vi "AO DM_WFS_master_v0.vi"() -> ()   [LabVIEW 2018]
uses:
  <userlib>/WaveKit.lib/Controls/Image information.ctl
  <userlib>/WaveKit.lib/Controls/Image general information.ctl
  <userlib>/WaveKit.lib/Controls/Image acquisition information.ctl
  <userlib>/WaveKit.lib/Controls/Point2D.ctl
  <userlib>/WaveKit.lib/Controls/Data alignment enum.ctl
  <userlib>/WaveKit.lib/Controls/StatisticsData.ctl
  <userlib>/WaveKit.lib/Controls/Wavefront Corrector states - ONE.ctl
  <userlib>/WaveKit.lib/Classes/Camera/Camera.lvclass
  <userlib>/WaveKit.lib/Classes/CameraSet/CameraSet.lvclass
  <userlib>/WaveKit.lib/Classes/Image/Image.lvclass
  <userlib>/WaveKit.lib/Classes/Phase/Phase.lvclass
  <userlib>/WaveKit.lib/Controls/HasoSlopes.lvclass
  <userlib>/WaveKit.lib/Controls/Pupil.lvclass
  <userlib>/WaveKit.lib/Classes/WavefrontCorrector/WavefrontCorrector.lvclass
  <userlib>/WaveKit.lib/Classes/WavefrontCorrectorSet/WavefrontCorrectorSet.lvclass
  <userlib>/WaveKit.lib/Classes/HasoEngine/HasoEngine.lvclass
  <userlib>/WaveKit.lib/Controls/SlopesEngineSetup.ctl
  <userlib>/WaveKit.lib/Controls/WavefrontReconstructionMode.ctl
  <vilib>/Utility/file.llb/Read From Spreadsheet File (DBL).vi
  <vilib>/Analysis/1siggen.llb/Ramp Pattern by Delta.vi
  <userlib>/WaveKit.lib/Classes/ModalCoef/ModalCoef.lvclass
  <vilib>/Analysis/NI_AALBase.lvlib
panel:
  in  "Device Status":enum32{"DM", "WFS", "Others"}(tab)
  out "DM Actuator Values":sgl[](graph)
  out "Initial State":T1[](array[typedef])
  out "ActuatorsNumber":i32
  out "Initial Positions":sgl[](array[numeric])
  out "Final Positions":sgl[](array[numeric])
  in  "Coef Min":dbl=-0.5 min=1.0
  in  "Coef Max":dbl=0.5 min=1.0
  out "Zernike Measured":dbl[](graph)
  out "Phase statistics":T2
  out "Phase values":sgl[][](graph)=[[nan, nan, nan, nan, nan, nan, nan, nan, nan, nan, nan, nan, nan, nan, nan, nan, nan, nan, nan, nan, nan, nan, nan, nan, nan, nan, nan, nan, nan, nan, nan, nan, nan, nan, nan, nan, nan, nan, nan, nan], [nan, nan, nan, nan, nan, nan, nan, nan, nan, nan, nan, nan, nan, nan, nan, nan, nan, nan, nan, nan, nan, nan, nan, nan, nan, nan, nan, nan, nan, nan, nan, nan, nan, nan, nan, nan, nan, nan, nan, nan], [nan, nan, nan, nan, nan, nan, nan, nan, nan, nan, nan, nan, nan, nan, nan, nan, nan, nan, nan, nan, nan, nan, nan, nan, nan, nan, nan, nan, nan, nan, nan, nan, nan, nan, nan, nan, nan, nan, nan, nan], [nan, nan, nan, nan, nan, nan, nan, nan, nan, nan, nan, nan, nan, nan, nan, nan, nan, nan, nan, nan, nan, nan, nan, nan, nan, nan, nan, nan, nan, nan, nan, nan, nan, nan, nan, nan, nan, nan, nan, nan], [nan, nan, nan, nan, nan, nan, nan, nan, nan, nan, nan, nan, nan, nan, -0.14441992, nan, 0.1501734, 0.22490476, 0.2674259, 0.28415325, 0.2792031, 0.2552752, 0.21375881, 0.15405469, nan, nan, nan, nan, nan, nan, nan, nan, nan, nan, nan, nan, nan, nan, nan, nan], [nan, nan, nan, nan, nan, nan, nan, nan, nan, nan, nan, nan, nan, nan, 0.19143742, 0.2795512, 0.33646506, 0.37099743, 0.3877919, 0.3894302, 0.37774685, 0.35447162, 0.3212538, 0.27904776, 0.22675864, 0.15897867, nan, nan, nan, nan, nan, nan, nan, nan, nan, nan, nan, nan, nan, nan], [nan, nan, nan, nan, nan, nan, nan, nan, nan, nan, nan, nan, nan, 0.22618562, 0.290776, 0.33285964, 0.36044422, 0.3767934, 0.38285175, 0.37884915, 0.3652757, 0.3433441, 0.3149789, 0.28229773, 0.2464756, 0.20580466, 0.15268901, 0.06923797, nan, nan, nan, nan, nan, nan, nan, nan, nan, nan, nan, nan], [nan, nan, nan, nan, nan, nan, nan, nan, nan, nan, nan, nan, 0.19992779, 0.24616541, 0.27565512, 0.29675642, 0.31222007, 0.32191983, 0.32467726, 0.31943765, 0.30597392, 0.2852214, 0.25927368, 0.2309889, 0.20308714, 0.17653626, 0.14795627, 0.10568966, 0.024115691, nan, nan, nan, nan, nan, nan, nan, nan, nan, nan, nan], [nan, nan, nan, nan, nan, nan, nan, nan, nan, nan, nan, 0.14862825, 0.18219855, 0.20114602, 0.21551609, 0.22862102, 0.24014233, 0.24817906, 0.2505626, 0.24567793, 0.23295718, 0.21313797, 0.18829979, 0.16161954, 0.1367108, 0.11633411, 0.10019377, 0.081457645, 0.04156301, -0.057204023, nan, nan, nan, nan, nan, nan, nan, nan, nan, nan], [nan, nan, nan, nan, nan, nan, nan, nan, nan, nan, 0.08899155, 0.117771566, 0.12948777, 0.13732892, 0.14631097, 0.15688494, 0.16728252, 0.17497937, 0.17758016, 0.17335457, 0.16157834, 0.14275661, 0.11873307, 0.09261118, 0.06834036, 0.04974218, 0.038678437, 0.031985473, 0.016725859, -0.03676957, nan, nan, nan, nan, nan, nan, nan, nan, nan, nan], [nan, nan, nan, nan, nan, nan, nan, nan, nan, nan, 0.058377307, 0.069048055, 0.0725615, 0.07683456, 0.0840318, 0.09335055, 0.10271386, 0.1097376, 0.11226265, 0.10867052, 0.09812171, 0.08078306, 0.058033932, 0.032565817, 0.008214329, -0.010712444, -0.020921554, -0.022825297, -0.02489755, -0.05023362, -0.14592764, nan, nan, nan, nan, nan, nan, nan, nan, nan], [nan, nan, nan, nan, nan, nan, nan, nan, nan, -0.0018393314, 0.018310271, 0.023098737, 0.024714457, 0.027986258, 0.033823933, 0.041292578, 0.048749834, 0.054400377, 0.056548227, 0.05374936, 0.04499338, 0.029967438, 0.009379062, -0.014759185, -0.03905803, -0.059140373, -0.070816256, -0.0724436, -0.06894927, -0.07806298, -0.1393881, nan, nan, nan, nan, nan, nan, nan, nan, nan], [nan, nan, nan, nan, nan, nan, nan, nan, nan, -0.03322208, -0.017045017, -0.0123043535, -0.010394985, -0.007970343, -0.0042642877, 0.0003761826, 0.005164365, 0.009095938, 0.010986101, 0.009512841, 0.0033822758, -0.008344227, -0.02579559, -0.047820807, -0.071688615, -0.09321856, -0.107681155, -0.11187886, -0.10789668, -0.10908524, -0.14891545, -0.29341945, nan, nan, nan, nan, nan, nan, nan, nan], [nan, nan, nan, nan, nan, nan, nan, nan, nan, nan, -0.043187555, -0.03622458, -0.033755217, -0.03278728, -0.03198469, -0.030707732, -0.028716512, -0.026208155, -0.023933899, -0.023217455, -0.025771504, -0.03328519, -0.04682974, -0.06620631, -0.08943447, -0.1126552, -0.13079928, -0.13944486, -0.13836564, -0.13734597, -0.16491348, -0.2807172, nan, nan, nan, nan, nan, nan, nan, nan], [nan, nan, nan, nan, nan, nan, nan, nan, -0.13038255, -0.08328184, -0.060542934, -0.050779276, -0.048053104, -0.048984695, -0.05126809, -0.053124577, -0.05330209, -0.051303368, -0.04760214, -0.04368073, -0.041799206, -0.04448101, -0.05377527, -0.07043236, -0.09320336, -0.118551016, -0.14113419, -0.15550357, -0.15952203, -0.16009864, -0.18189941, -0.27977645, nan, nan, nan, nan, nan, nan, nan, nan], [nan, nan, nan, nan, nan, nan, nan, nan, -0.15416794, -0.09987456, -0.07151361, -0.05893044, -0.056102008, -0.058817875, -0.063637674, -0.067669004, -0.06878706, -0.06599128, -0.059670344, -0.051622536, -0.044753395, -0.042448726, -0.04769562, -0.062100213, -0.08502676, -0.11315687, -0.14084403, -0.16171429, -0.1720384, -0.17647736, -0.19687745, -0.284868, -0.53908885, -1.12795, nan, nan, nan, nan, nan, nan], [nan, nan, nan, nan, nan, nan, nan, nan, -0.17633308, -0.1131372, -0.07876157, -0.06330658, -0.060116876, -0.063924976, -0.07015394, -0.07493687, -0.07548633, -0.07052183, -0.060539607, -0.047784284, -0.035856243, -0.028966732, -0.030924596, -0.044017438, -0.06802279, -0.099662215, -0.13288532, -0.16044727, -0.17731819, -0.18653797, -0.20820689, -0.29237592, -0.5366785, nan, nan, nan, nan, nan, nan, nan], [nan, nan, nan, nan, nan, nan, nan, nan, -0.19826387, -0.12505035, -0.08430402, -0.06564974, -0.061443567, -0.06527472, -0.07152294, -0.07554153, -0.07411167, -0.0658889, -0.05163869, -0.034133032, -0.017655006, -0.0071354215, -0.007018423, -0.020031396, -0.046107426, -0.08178567, -0.12048963, -0.15415914, -0.17678727, -0.19048853, -0.21480094, -0.2999987, -0.54526997, nan, nan, nan, nan, nan, nan, nan], [nan, nan, nan, nan, nan, nan, nan, nan, -0.2214154, -0.13693352, -0.08914254, -0.06661926, -0.06048554, -0.06317037, -0.0681367, -0.07015528, -0.065784656, -0.053790003, -0.035310905, -0.013662348, 0.0062713036, 0.01901285, 0.01972933, 0.005542416, -0.023349542, -0.06307545, -0.10643376, -0.14466219, -0.17119798, -0.18806857, -0.21562657, -0.30642, -0.5640642, nan, nan, nan, nan, nan, nan, nan], [nan, nan, nan, nan, nan, nan, nan, nan, -0.24718054, -0.14940841, -0.093277775, -0.0658183, -0.056708053, -0.05720259, -0.059951056, -0.05929426, -0.051715773, -0.036192447, -0.014265999, 0.010266874, 0.032073133, 0.04536258, 0.04520398, 0.028878966, -0.0030008797, -0.045963787, -0.092160165, -0.13235793, -0.16002774, -0.17817038, -0.20961209, -0.31157303, -0.5953845, nan, nan, nan, nan, nan, nan, nan], [nan, nan, nan, nan, nan, nan, nan, nan, -0.27748746, -0.16290864, -0.09610232, -0.062047683, -0.048735943, -0.04617936, -0.046241976, -0.042900223, -0.03261665, -0.014586102, 0.009311387, 0.03494107, 0.05674191, 0.068891875, 0.0666744, 0.04783368, 0.0136316735, -0.030755527, -0.0769404, -0.115639456, -0.14119013, -0.15893419, -0.19620675, -0.31774768, nan, nan, nan, nan, nan, nan, nan, nan], [nan, nan, nan, nan, nan, nan, nan, nan, -0.31623095, -0.17884897, -0.09729818, -0.0539262, -0.03469713, -0.028198741, -0.025418447, -0.019910373, -0.008048305, 0.010862423, 0.034768496, 0.05942371, 0.07931873, 0.0889112, 0.08400761, 0.06307276, 0.028166434, -0.014867521, -0.057410896, -0.09080534, -0.111413695, -0.12868427, -0.17697167, -0.3319423, nan, nan, nan, nan, nan, nan, nan, nan], [nan, nan, nan, nan, nan, nan, nan, nan, nan, -0.20170604, -0.09850275, -0.0411539, -0.0131010795, -0.0011654077, 0.0047943285, 0.01185911, 0.023955166, 0.041901454, 0.06374147, 0.08542206, 0.1018104, 0.10796184, 0.10047772, 0.0787158, 0.04554086, 0.007227666, -0.027947046, -0.052963093, -0.06777905, -0.08820889, -0.15871821, nan, nan, nan, nan, nan, nan, nan, nan, nan], [nan, nan, nan, nan, nan, nan, nan, nan, nan, -0.24239759, -0.10614249, -0.026831074, 0.015322472, 0.03581071, 0.046350636, 0.05505173, 0.06651187, 0.08204405, 0.10016226, 0.11737824, 0.12928592, 0.13183476, 0.12261822, 0.10192663, 0.073240966, 0.042765103, 0.017522467, 0.0014635092, -0.0110412, -0.045025453, -0.15884721, nan, nan, nan, nan, nan, nan, nan, nan, nan], [nan, nan, nan, nan, nan, nan, nan, nan, nan, nan, -0.13597216, -0.021381527, 0.04426403, 0.07956008, 0.09847209, 0.110732496, 0.122154154, 0.13505057, 0.14887714, 0.16113368, 0.16849175, 0.16803522, 0.1584293, 0.14075197, 0.118653886, 0.09743117, 0.0815231, 0.06987105, 0.048498146, -0.020404778, nan, nan, nan, nan, nan, nan, nan, nan, nan, nan], [nan, nan, nan, nan, nan, nan, nan, nan, nan, nan, nan, -0.04876471, 0.05625415, 0.117832564, 0.15310521, 0.17423762, 0.18897903, 0.20128381, 0.21210447, 0.22038196, 0.22418612, 0.221881, 0.21311647, 0.19937092, 0.1836943, 0.16922635, 0.15598845, 0.13537171, 0.081669986, nan, nan, nan, nan, nan, nan, nan, nan, nan, nan, nan], [nan, nan, nan, nan, nan, nan, nan, nan, nan, nan, nan, nan, 0.014031529, 0.121263236, 0.18738765, 0.22803904, 0.25380248, 0.2710389, 0.28282017, 0.2899857, 0.29225817, 0.2892868, 0.28139976, 0.26978248, 0.25571787, 0.23844866, 0.21115, 0.15442081, nan, nan, nan, nan, nan, nan, nan, nan, nan, nan, nan, nan], [nan, nan, nan, nan, nan, nan, nan, nan, nan, nan, nan, nan, nan, nan, 0.15212902, 0.2306162, 0.28129596, 0.31381333, 0.33402625, 0.3450995, 0.34855807, 0.34515002, 0.33529556, 0.31882071, 0.29360068, 0.25266168, nan, nan, nan, nan, nan, nan, nan, nan, nan, nan, nan, nan, nan, nan], [nan, nan, nan, nan, nan, nan, nan, nan, nan, nan, nan, nan, nan, nan, nan, nan, 0.1979487, 0.2623494, 0.30271748, 0.32490522, 0.33223343, 0.3261181, 0.30614072, 0.26925305, nan, nan, nan, nan, nan, nan, nan, nan, nan, nan, nan, nan, nan, nan, nan, nan], [nan, nan, nan, nan, nan, nan, nan, nan, nan, nan, nan, nan, nan, nan, nan, nan, nan, nan, nan, nan, nan, nan, nan, nan, nan, nan, nan, nan, nan, nan, nan, nan, nan, nan, nan, nan, nan, nan, nan, nan], [nan, nan, nan, nan, nan, nan, nan, nan, nan, nan, nan, nan, nan, nan, nan, nan, nan, nan, nan, nan, nan, nan, nan, nan, nan, nan, nan, nan, nan, nan, nan, nan, nan, nan, nan, nan, nan, nan, nan, nan], [nan, nan, nan, nan, nan, nan, nan, nan, nan, nan, nan, nan, nan, nan, nan, nan, nan, nan, nan, nan, nan, nan, nan, nan, nan, nan, nan, nan, nan, nan, nan, nan, nan, nan, nan, nan, nan, nan, nan, nan]] caption="Wavefront"
  out "HASO intensity":u32[][](graph)
  out "Current error":errorcluster
  out "Output path":path=path "D:/Data"
  in  "Current status":string="Test1"
  out "HASO ready":bool
  in  "Live Wavefront":bool
  in  "Update DM":bool
  in  "Tab Control":T3(tab)
  in  "Initial haso file":path=path "D:/SystemAlignment/system_aberration_residual_20200816.has"
  in  "interaction matrix file":path=path "D:/SystemAlignment/IM_20200807_1p5s.aomi"
  in  "DM configuration file":path=path "C:/Program Files (x86)/Imagine Optic/Configuration Files/WaveFrontCorrector_mirao52-e_0326.dat"
  in  "Haso configuration file":path=path "C:/Program Files (x86)/Imagine Optic/Configuration Files/HASO3_first_7364.dat"
  in  "Coef value":dbl=0.5 min=1.0
  in  "Idx end":u32=20 min=1
  in  "Idx start":u32=1 min=1
  in  "Subfolder":string="Test1"
  in  "Folder Name":string="Test"
  in  "Record Response":bool
  in  "Net Rp":bool
  in  "Input type":T4(ring)=enum."Zernike Coef"
  in  "Additional Command":bool=TRUE
  in  "Offset command file":path=path "D:/SystemAlignment/system_aberration_20200627.dat"
  in  "Initial offset":bool=TRUE
  in  "Additional file":path=path "D:/SystemAlignment/system_aberration_20191029.dat"
  out "Zern coef out":sgl[](array[numeric])
  out "Zern index out":i32[](array[numeric])
  in  "Zern index in":i32[](array[numeric])
  in  "Zern coef in":sgl[](array[numeric])
  in  "idxType":enum16{"Wyant", "ANSI"}(ring)
  in  "Filter":u8[](array[numeric])
  out "exposure_duration_us (get)":u32
  in  "exposure_duration_s (set)":dbl=0.5 min=1.0
  out "nb_images (get)":u32=10
  in  "nb_images (set)":u32=1 min=1
  in  "Save File":bool
  in  "File Base Name":string="Test"
  in  "Main Path":path=path "D:/Data"
  in  "Record Batch":bool
  out "Acquisition information":T5={"Image general information"={"Camera serial number"="", "Smearing removed"=FALSE, "Background image removed"=FALSE, "Time Stamp"=timestamp(0 s since 1904-01-01), "Comment"="", "Camera_MAX_Level"=0}, "Acquisition information"={"Exposure duration (us)"=0, "Exposure duration specified (us)"=0, "Gain"=0.0, "Number of summed images"=0, "Trigger type"=""}, "Number of pixels"={"X"=0, "Y"=0}, "Number of bits"=enum."16"}
  in  "Init":bool
  in  "Reset error":bool
  in  "Exit":bool
  in  "Stop HASO":bool
  in  "Start HASO":bool
  # "AO DM_WFS_master_v0.vi: (last update: 20200817)\nControl deformable mirror and wavefront sensor, check DM response be WFS \n1, Record DM response;\n2, Test DM response to single Zernike component in batch"
  # "um"
  # "HASO Parameters"
  # "Check DM Response"
  # "Need to turn OFF live wavefront"
  # "Batch range"
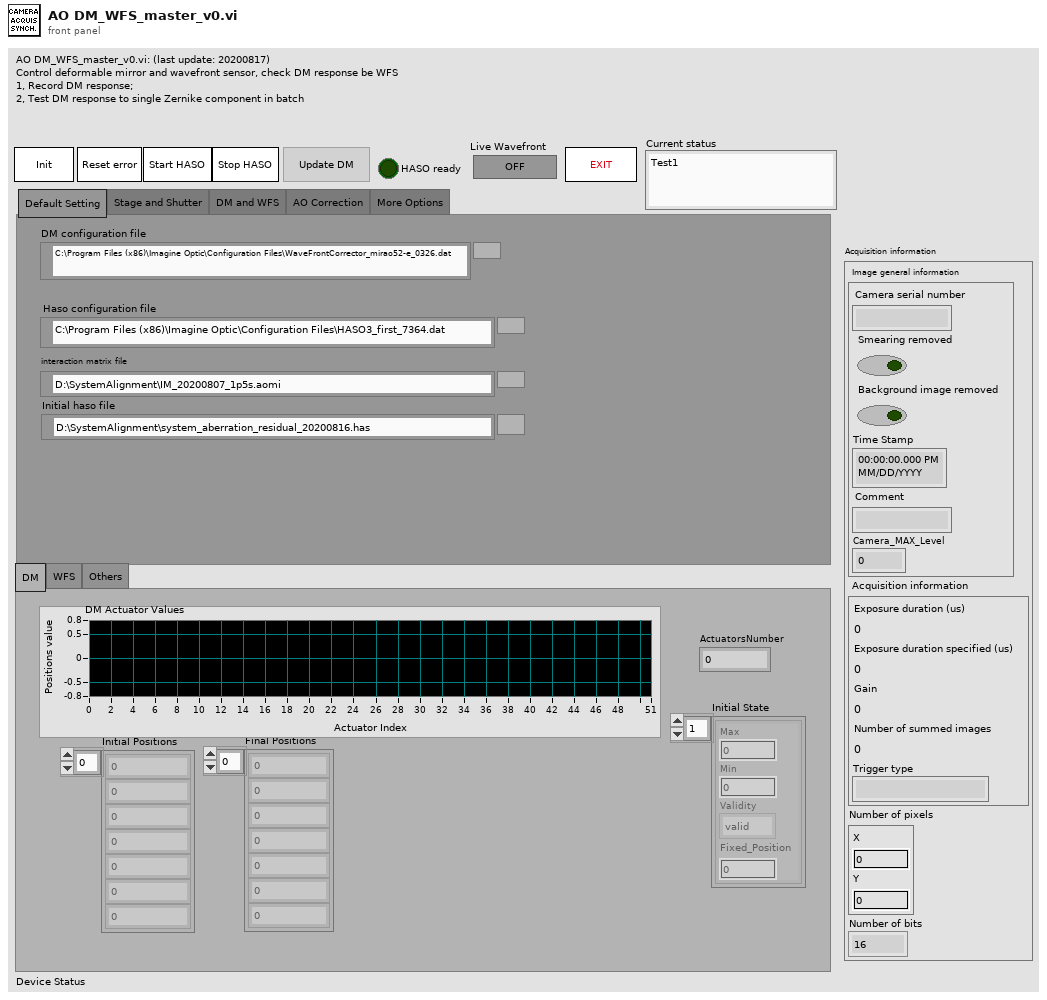
[diagram p1: front panel]
types:
  T1 = typedef "Wavefront Corrector states - ONE.ctl" = cluster{"Max":sgl, "Min":sgl, "Validity":enum16{"valid", "fixed", "invalid"}, "Fixed_Position":sgl}
  T2 = typedef "StatisticsData.ctl" = cluster{"PV":sgl, "RMS":dbl, "Max":sgl, "Min":sgl}
  T3 = enum32{"Default Setting", "Stage and Shutter", "DM and WFS", "AO Correction", "More Options"}
  T4 = enum16{"Zero Input", "Command File", "Zernike Coef", "Zernike File"}
  T5 = typedef "Image information.ctl" = cluster{"Image general information":T6, "Acquisition information":T7, "Number of pixels":T8, "Number of bits":T9}
  T6 = typedef "Image general information.ctl" = cluster{"Camera serial number":string, "Smearing removed":bool, "Background image removed":bool, "Time Stamp":timestamp, "Comment":string, "Camera_MAX_Level":i32}
  T7 = typedef "Image acquisition information.ctl" = cluster{"Exposure duration (us)":i32, "Exposure duration specified (us)":i32, "Gain":sgl, "Number of summed images":i32, "Trigger type":string}
  T8 = typedef "Point2D.ctl" = cluster{"X":u32, "Y":u32}
  T9 = typedef "Data alignment enum.ctl" = enum16{"8", "16", "32"}
  T10 = typedef "SlopesEngineSetup.ctl" = cluster{"Start sub-aperture":T8, "Pupil average":dbl}
  T11 = typedef "CameraSpecifications.ctl" = cluster{"Grabber name":string, "Camera name":string, "Camera sn":string, "Pixels_um":T12, "Maximum level":u32, "Data alignment":T9, "Is signed":bool, "Acquisition start":T8, "Acquisition length":T8, "MaxFrameRate_Hz":sgl, "Chip type":enum16{"Progressive scan", "Frame transfert"}}
  T12 = typedef "General dimensions definition.ctl" = cluster{"Size":T8, "Step":T13}
  T13 = typedef "Point2Df.ctl" = cluster{"X":sgl, "Y":sgl}
  T14 = typedef "Wavefront Corrector Position.ctl" = sgl[]
  T15 = typedef "WavefrontReconstructionMode.ctl" = enum16{"None", "Modal_Legendre", "Modal_Zernike", "Zonal", "Modal_Zonal_Zernike", "Modal_Zonal_Legendre"}
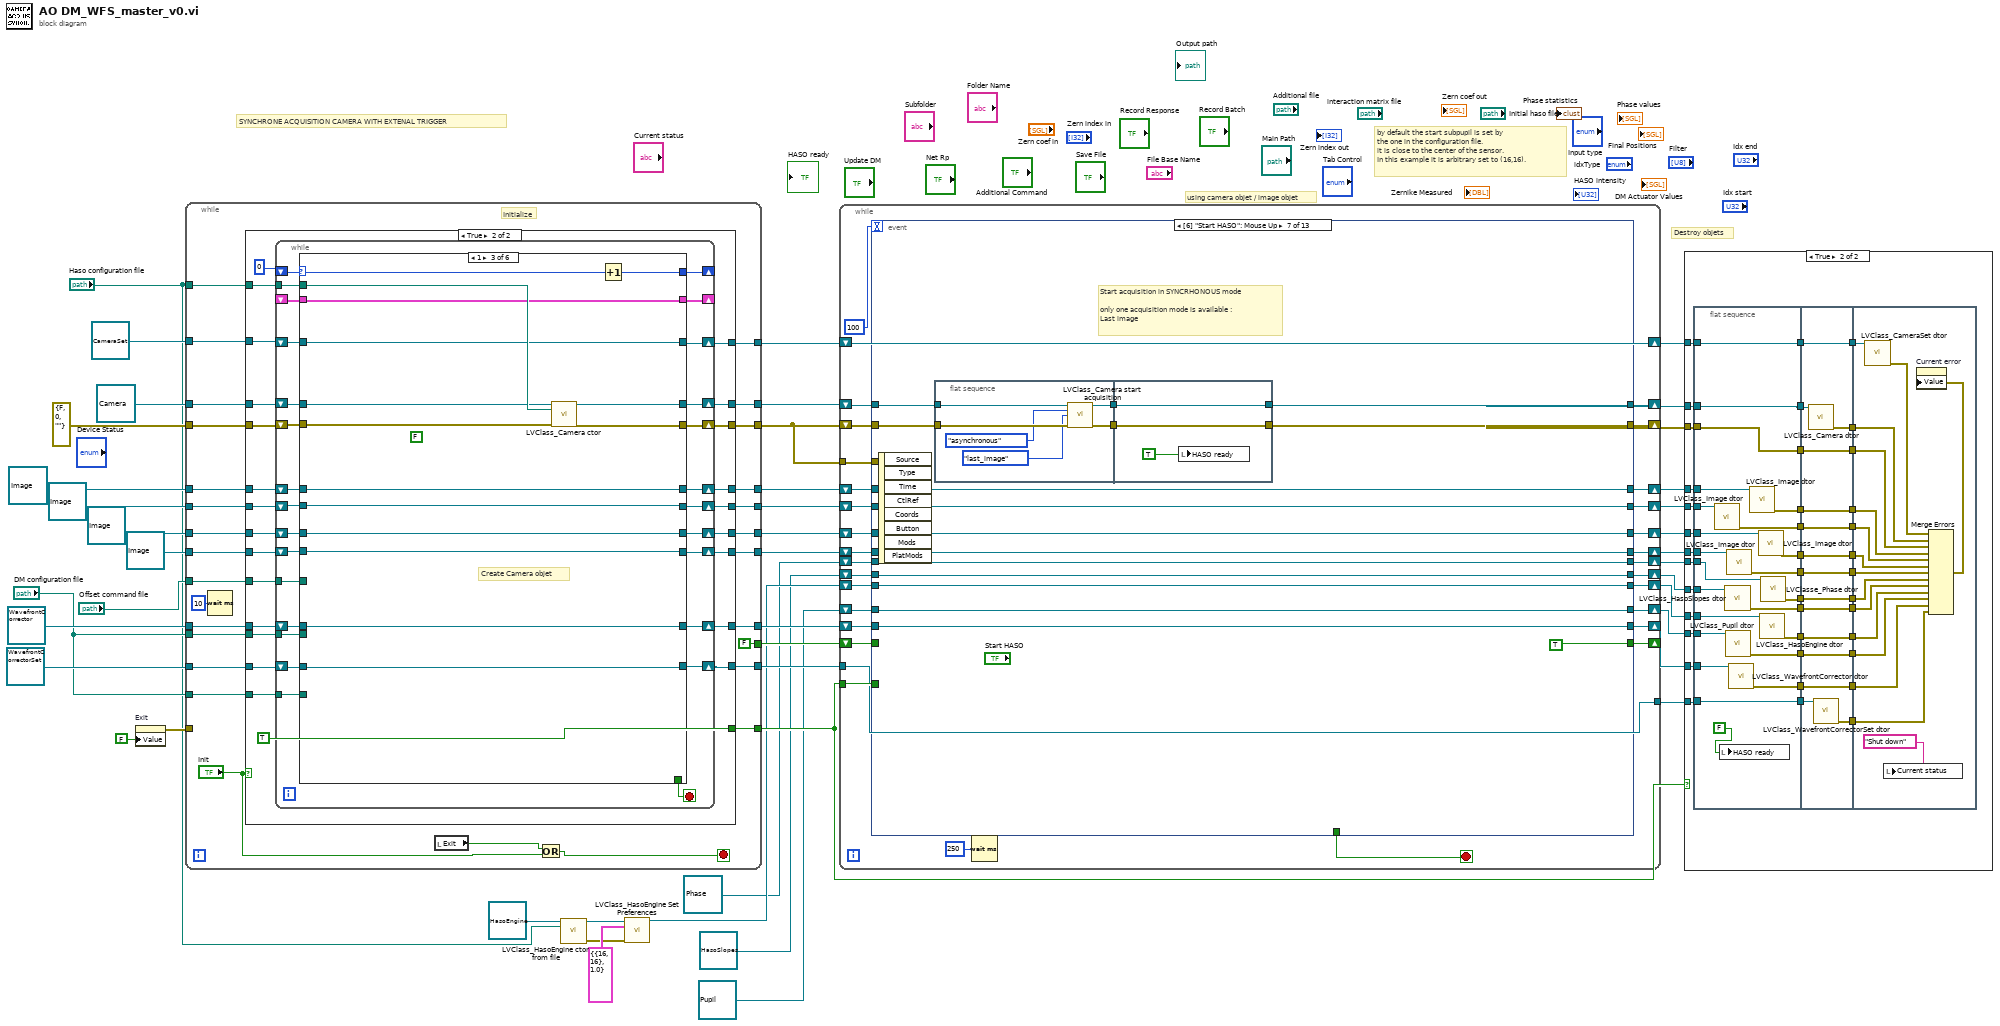
[diagram p0: block diagram]
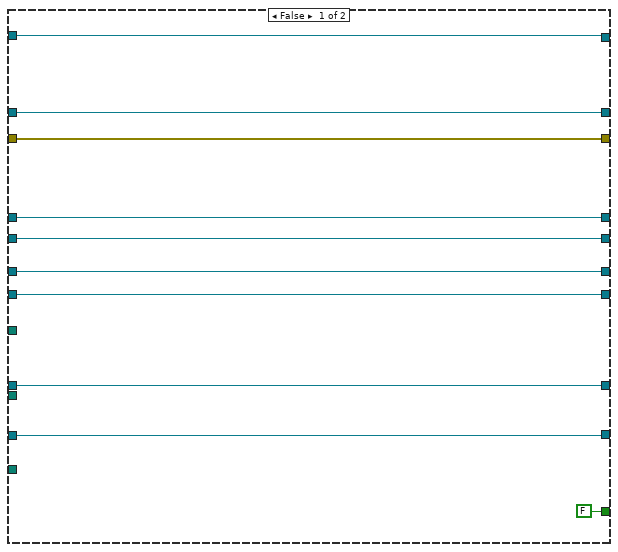
[diagram p3: hidden frame]
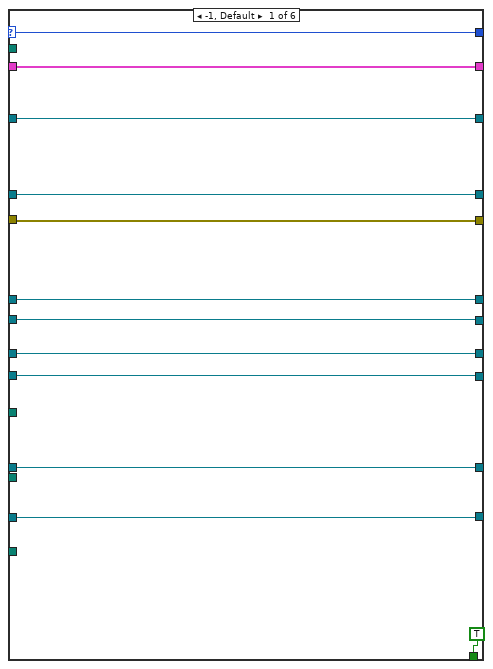
[diagram p4: hidden frame]
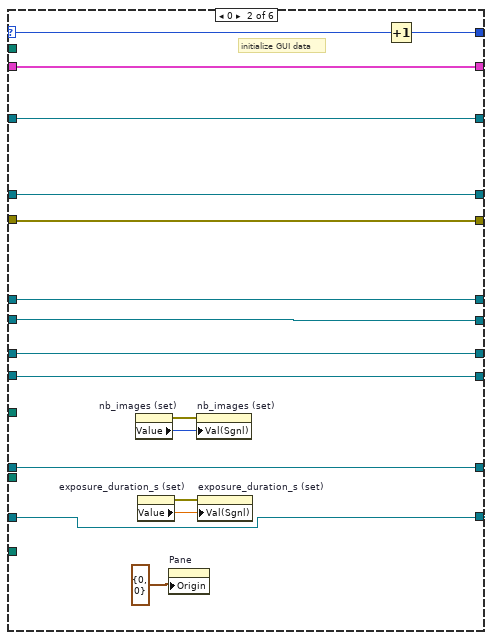
[diagram p5: hidden frame]
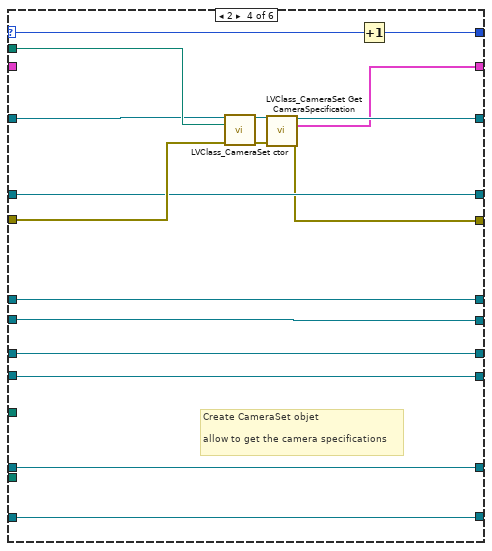
[diagram p6: hidden frame]
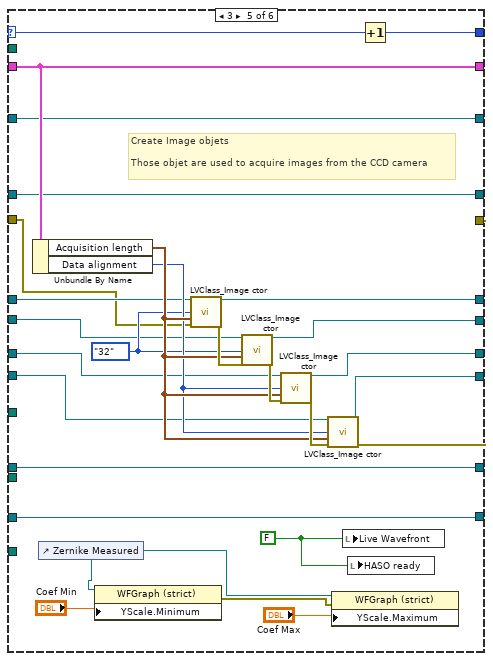
[diagram p7: hidden frame]
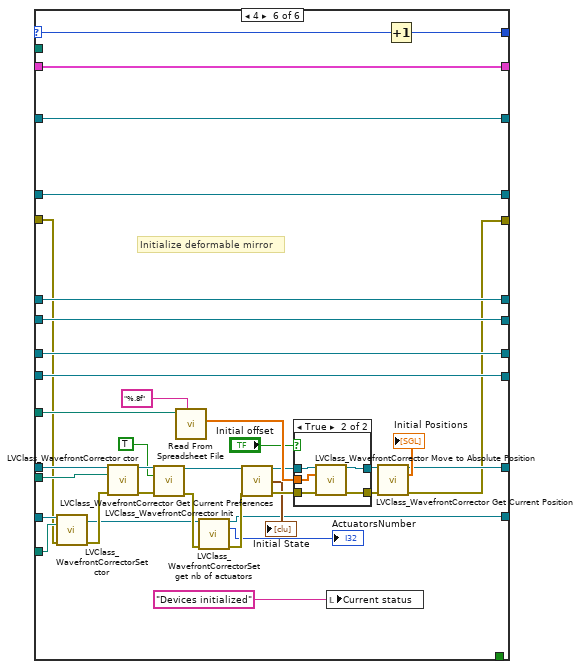
[diagram p8: hidden frame]
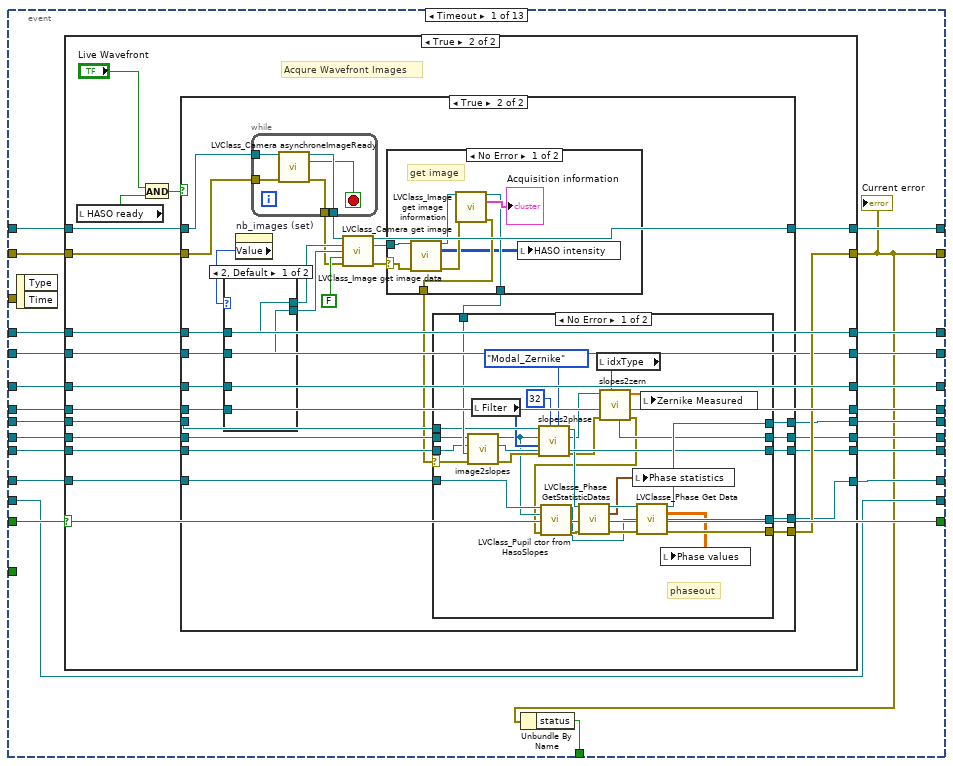
[diagram p10: hidden frame]
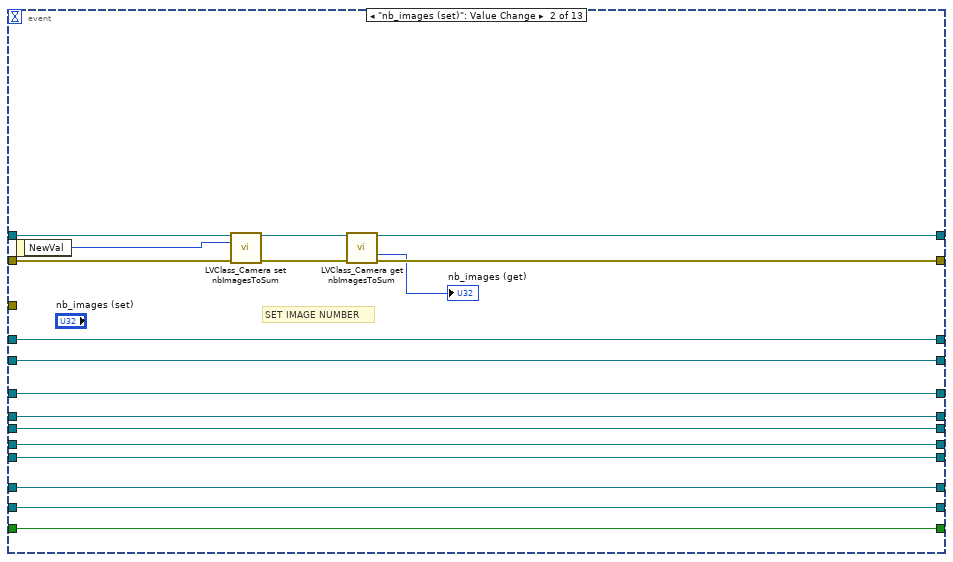
[diagram p16: hidden frame]
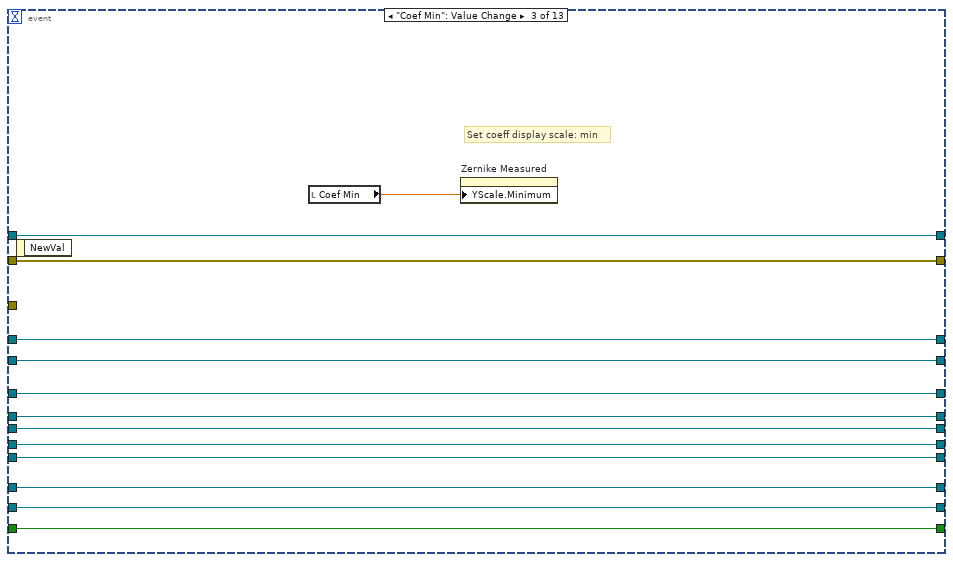
[diagram p17: hidden frame]
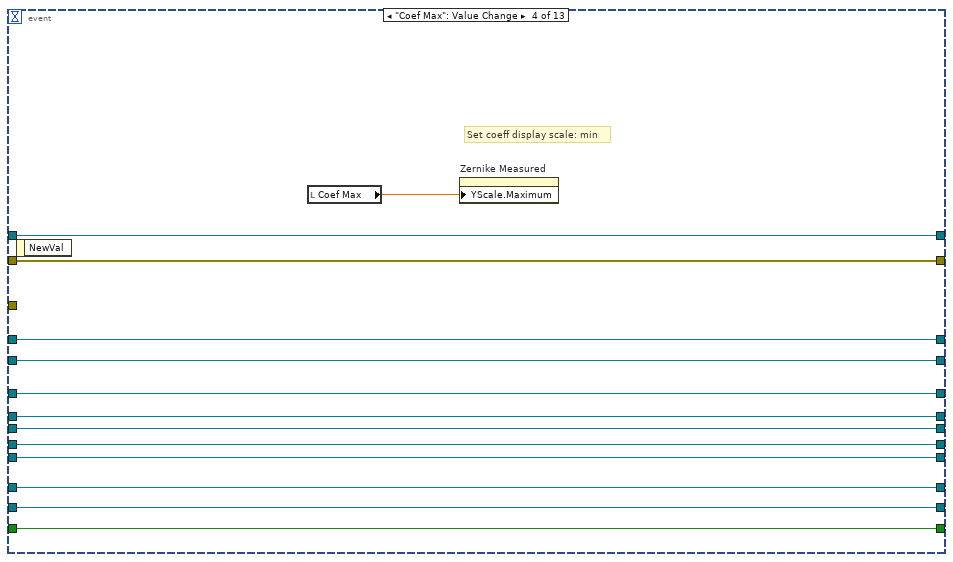
[diagram p18: hidden frame]
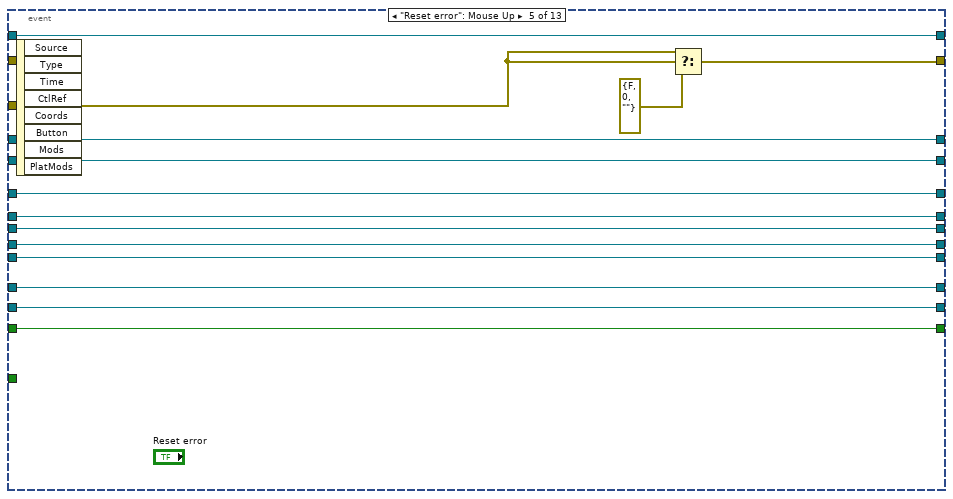
[diagram p19: hidden frame]
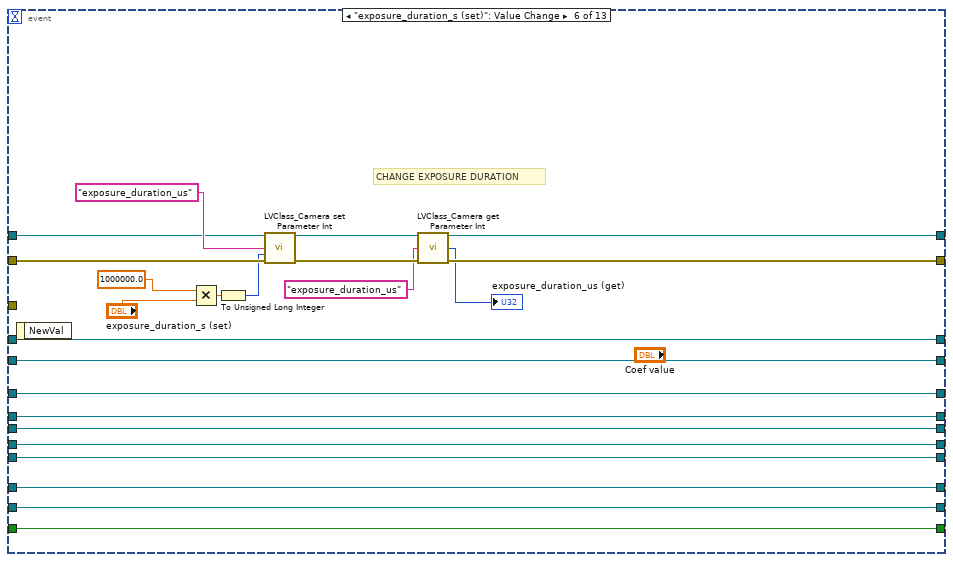
[diagram p20: hidden frame]
diagram:
  # "by default the start subpupil is set by \nthe one in the configuration file. \nit is close to the center of the sensor.\nIn this example it is arbitrary set to (16,16)."
  # "Destroy objets"
  # "using camera objet / image objet"
  # "SYNCHRONE ACQUISITION CAMERA WITH EXTENAL TRIGGER"
  n1 = property on="Exit" class="Bool (strict)"("Value"=FALSE ("Exit")) -> (error out=w22:errorcluster)  [unwired: 2 in, 1 out]
  n2 = while {
    tunnel: [FALSE] -> w39
    tunnel: [w73] -> w38
    tunnel: [w72] -> w37
    tunnel: [w71] -> w36
    tunnel: [w70] -> w35
    tunnel: [w69] -> w34
    tunnel: [w68] -> w33
    tunnel: refnum<class "Camera.lvclass"> refnum ("Camera.lvclass") -> [w67]
    tunnel: refnum<class "CameraSet.lvclass"> refnum ("CameraSet.lvclass") -> [w66]
    tunnel: refnum<class "Image.lvclass"> refnum ("Image in") -> [w65]
    tunnel: refnum<class "Image.lvclass"> refnum ("Image in") -> [w64]
    tunnel: refnum<class "Image.lvclass"> refnum ("Image in") -> [w63]
    tunnel: refnum<class "Image.lvclass"> refnum ("Image in") -> [w62]
    tunnel: errorcluster {"status"=FALSE, "code"=0, "source"=""} ("error out") -> [w61]
    tunnel: [w60] -> w25
    tunnel: [w58] -> w24
    tunnel: w22 -> [_]
    tunnel: "Haso configuration file" -> [w54]
    tunnel: "Offset command file" -> [w53]
    tunnel: refnum<class "WavefrontCorrectorSet.lvclass"> refnum ("WavefrontCorrectorSet in") -> [w52]
    tunnel: "DM configuration file" -> [w51]
    tunnel: refnum<class "WavefrontCorrector.lvclass"> refnum ("WavefrontCorrector in") -> [w50]
    tunnel: "DM configuration file" -> [w49]
    tunnel: [w48] -> w17
    tunnel: [w47] -> w16
    stop <- w55 stop-if-true
    # "Initialize"
    n3 = Wait (ms)(milliseconds to wait=u32 10) -> ()  [unwired: 1 out]
    n4 = case shown="True" "Init" {
      tunnel: [w84 w108] -> w73
      tunnel: [w83 w107] -> w72
      tunnel: [w81 w106] -> w71
      tunnel: [w80 w105] -> w70
      tunnel: [w79 w104] -> w69
      tunnel: [w78 w103] -> w68
      tunnel: w67 -> [w84 w102]
      tunnel: w66 -> [w83 w100]
      tunnel: w65 -> [w81 w99]
      tunnel: w64 -> [w80 w98]
      tunnel: w63 -> [w79 w97]
      tunnel: w62 -> [w78 w96]
      tunnel: w61 -> [w82 w95]
      tunnel: [w82 w94] -> w60
      tunnel: [FALSE TRUE] -> w58
      tunnel: w54 -> [_ w92]
      tunnel: w53 -> [_ w91]
      tunnel: w52 -> [w75 w85]
      tunnel: w51 -> [_ w90]
      tunnel: w50 -> [w76 w86]
      tunnel: w49 -> [_ w89]
      tunnel: [w76 w88] -> w48
      tunnel: [w75 w87] -> w47
      frame False {
      }
      frame True {
        n5 = while {
          tunnel: w92 -> [w133]
          shift-right: [w135] -> w108
          shift-left: w102 -> [w127]
          shift-right: [w117] -> _
          shift-left: 0 -> [w116]
          shift-right: [w134] -> w107
          shift-left: w100 -> [w126]
          shift-right: [w125] -> _
          shift-left: _ -> [w123]
          shift-right: [w132] -> w106
          shift-left: w99 -> [w124]
          shift-right: [w131] -> w105
          shift-left: w98 -> [w122]
          shift-right: [w130] -> w104
          shift-left: w97 -> [w120]
          shift-right: [w129] -> w103
          shift-left: w96 -> [w121]
          shift-right: [w128] -> w94
          shift-left: w95 -> [w118]
          tunnel: w91 -> [w115]
          tunnel: w90 -> [w114]
          tunnel: w89 -> [w113]
          shift-right: [w112] -> w88
          shift-left: w86 -> [w110]
          shift-right: [w111] -> w87
          shift-left: w85 -> [w109]
          stop <- w119 stop-if-true
          n6 = case shown="1" w116 {
            tunnel: [w147 w151 w179 w189 w211 w261] -> w135
            tunnel: w133 -> [_ _ w178 w193 _ _]
            tunnel: [w146 w155 w176 w194 w212 w260] -> w134
            tunnel: [w139 w156 w170 w184 w218 w255] -> w132
            tunnel: [w140 w157 w171 w185 w217 w256] -> w131
            tunnel: [w141 w158 w172 w186 w216 w257] -> w130
            tunnel: [w142 w159 w173 w187 w215 w258] -> w129
            tunnel: [w143 w150 w175 w188 w214 w229] -> w128
            selector: w116 -> [w138 w153 w168 w183 w206 w227]
            tunnel: w127 -> [w147 w151 w177 w189 w211 w261]
            tunnel: w126 -> [w146 w155 w176 w192 w212 w260]
            tunnel: [w144 w152 w174 w191 w213 w259] -> w125
            tunnel: w124 -> [w139 w156 w170 w184 w210 w255]
            tunnel: w123 -> [w144 w152 w174 _ w213 w259]
            tunnel: w122 -> [w140 w157 w171 w185 w209 w256]
            tunnel: w121 -> [w142 w159 w173 w187 w208 w258]
            tunnel: w120 -> [w141 w158 w172 w186 w207 w257]
            tunnel: [TRUE _ _ _ _ _] -> w119
            tunnel: w118 -> [w143 w150 w167 w190 w204 w230]
            tunnel: [w138 w154 w169 w182 w205 w226] -> w117
            tunnel: w115 -> [_ _ _ _ _ w237]
            tunnel: w109 -> [w136 w148 w165 w180 w202 w235]
            tunnel: w114 -> [_ _ _ _ _ w234]
            tunnel: w110 -> [w137 w149 w166 w181 w203 w233]
            tunnel: w113 -> [_ _ _ _ _ w232]
            tunnel: [w137 w149 w166 w181 w203 w231] -> w112
            tunnel: [w136 w148 w165 w180 w202 w228] -> w111
            frame -1, Default {
            }
            frame 0 {
              # "initialize GUI data"
              n7 = property on="nb_images (set)" class="DigNum (strict)"() -> (error out=w164:errorcluster, "Value"=w163:u32)  [unwired: 2 in, 1 out]
              n8 = property on="exposure_duration_s (set)" class="DigNum (strict)"() -> (error out=w160:errorcluster, "Value"=w162:dbl)  [unwired: 2 in, 1 out]
              n9 = property on="Pane" class="Pane"("Origin"=cluster{"Horizontal":i16, "Vertical":i16} {"Horizontal"=0, "Vertical"=0} ("Front Panel Window:Origin")) -> ()  [unwired: 2 in, 2 out]
              n10 = property on="nb_images (set)" class="DigNum (strict)"(error in=w164, "Val(Sgnl)"=w163) -> ()  [unwired: 1 in, 2 out]
              n11 = property on="exposure_duration_s (set)" class="DigNum (strict)"(error in=w160, "Val(Sgnl)"=w162) -> ()  [unwired: 1 in, 2 out]
              n12 = Increment(x=w153) -> (x+1=w154:i32)
            }
            frame 1 {
              (unwired) FALSE ("Acq required")
              # "Create Camera objet"
              n13 = call <userlib>:"LVClass_Camera ctor.vi"("Camera"=w177, "Configuration file path"=w178, "error in (no error)"=w167) -> ("Camera (new)"=w179:refnum<class "Camera.lvclass">, "error out"=w175:errorcluster)  [unwired: 11 in]
              n14 = Increment(x=w168) -> (x+1=w169:i32)
            }
            frame 2 {
              # "Create CameraSet objet\n\nallow to get the camera specifications"
              n15 = call <userlib>:"LVClass_CameraSet ctor.vi"("CameraSet.lvclass"=w192, "Configuration file path"=w193, "error in (no error)"=w190) -> ("CameraSet.lvclass"=w196:refnum<class "CameraSet.lvclass">, "error out"=w195:errorcluster)  [unwired: 11 in]
              n16 = call <userlib>:"LVClass_CameraSet Get CameraSpecification.vi"("CameraSet.lvclass"=w196, "error in (no error)"=w195) -> ("CameraSet.lvclass"=w194:refnum<class "CameraSet.lvclass">, "Camera Config"=w191:T11, "error out"=w188:errorcluster)  [unwired: 11 in]
              n17 = Increment(x=w183) -> (x+1=w182:i32)
            }
            frame 3 {
              w201 = FALSE
              w219 = Data_alignment_enum."32" ("Data alignment")
              # "Create Image objets\n\nThose objet are used to acquire images from the CCD camera"
              n18 = Unbundle By Name(w213) -> ("Acquisition length"=w221:T8, "Data alignment"=w220:T9)
              n19 = control-ref of="Zernike Measured"() -> (w198:refnum<vi>)
              n20 = property on="Property Node" class="WFGraph (strict)"(reference=w198, "YScale.Minimum"="Coef Min") -> (error out=w197:errorcluster)  [unwired: 1 in, 1 out]
              n21 = call <userlib>:"LVClass_Image ctor.vi"("Image in"=w210, "Data alignment"=w219, "Size"=w221, "error in (no error)"=w204) -> ("Image out"=w218:refnum<class "Image.lvclass">, "error out"=w222:errorcluster)  [unwired: 10 in]
              n22 = call <userlib>:"LVClass_Image ctor.vi"("Image in"=w209, "Data alignment"=w219, "Size"=w221, "error in (no error)"=w222) -> ("Image out"=w217:refnum<class "Image.lvclass">, "error out"=w223:errorcluster)  [unwired: 10 in]
              n23 = call <userlib>:"LVClass_Image ctor.vi"("Image in"=w207, "Data alignment"=w220, "Size"=w221, "error in (no error)"=w223) -> ("Image out"=w216:refnum<class "Image.lvclass">, "error out"=w224:errorcluster)  [unwired: 10 in]
              n24 = call <userlib>:"LVClass_Image ctor.vi"("Image in"=w208, "Data alignment"=w220, "Size"=w221, "error in (no error)"=w224) -> ("Image out"=w215:refnum<class "Image.lvclass">, "error out"=w214:errorcluster)  [unwired: 10 in]
              n25 = property on="Property Node" class="WFGraph (strict)"(reference=w198, error in=w197, "YScale.Maximum"="Coef Max") -> ()  [unwired: 2 out]
              n26 = local write "Live Wavefront"(w201) -> ()
              n27 = local write "HASO ready"(w201) -> ()
              n28 = Increment(x=w206) -> (x+1=w205:i32)
            }
            frame 4 {
              (unwired) "DM "
              (unwired) "DM "
              # "Initialize deformable mirror"
              n29 = call <userlib>:"LVClass_WavefrontCorrectorSet ctor.vi"("WavefrontCorrectorSet in"=w235, "PathToWavefrontCorrectorSetupFile"=w234, "error in (no error)"=w230) -> ("WavefrontCorrectorSet out"=w242:refnum<class "WavefrontCorrectorSet.lvclass">, "error out"=w251:errorcluster)  [unwired: 11 in]
              n30 = call <userlib>:"LVClass_WavefrontCorrector ctor.vi"("WavefrontCorrector in"=w233, "PathToWavefrontCorrectorSetupFile"=w232, "error in (no error)"=w251) -> ("WavefrontCorrector out"=w239:refnum<class "WavefrontCorrector.lvclass">, "error out"=w240:errorcluster)  [unwired: 11 in]
              n31 = call <userlib>:"LVClass_WavefrontCorrector Init.vi"("WavefrontCorrector in"=w239, "set_init_state_from_config_file"=TRUE, "error in (no error)"=w240) -> ("WavefrontCorrector out"=w243:refnum<class "WavefrontCorrector.lvclass">, "error out"=w252:errorcluster)  [unwired: 11 in]
              n32 = call-poly <vilib>:"Read From Spreadsheet File.vi"("format (%.3f)"="%.8f", "file path (dialog if empty)"=w237) -> ("first row"=w254:dbl[])  [unwired: 5 in, 4 out]
              n33 = call <userlib>:"LVClass_WavefrontCorrectorSet get nb of actuators.vi"("WavefrontCorrectorSet in"=w242, "error in (no error)"=w252) -> ("WavefrontCorrectorSet out"=w228:refnum<class "WavefrontCorrectorSet.lvclass">, "ActuatorsNumber"=→"ActuatorsNumber":i32, "error out"=w253:errorcluster)  [unwired: 11 in]
              n34 = call <userlib>:"LVClass_WavefrontCorrector Get Current Preferences.vi"("WavefrontCorrector in"=w243, "error in (no error)"=w253) -> ("WavefrontCorrector out"=w248:refnum<class "WavefrontCorrector.lvclass">, "Mirror preferences.Wavefront Corrector State"=→"Initial State":T1[], "error out"=w249:errorcluster)  [unwired: 10 in, 1 out]
              n35 = case shown="True" "Initial offset" {
                tunnel: w254 -> [_ w268]
                tunnel: [w263 w267] -> w246
                tunnel: [w262 w266] -> w247
                tunnel: w248 -> [w263 w265]
                tunnel: w249 -> [w262 w264]
                frame False {
                }
                frame True {
                  n36 = call <userlib>:"LVClass_WavefrontCorrector Move to Absolute Position.vi"("WavefrontCorrector in"=w265, "Absolute Positions"=w268, "error in (no error)"=w264) -> ("WavefrontCorrector out"=w267:refnum<class "WavefrontCorrector.lvclass">, "error out"=w266:errorcluster)  [unwired: 11 in]
                }
              }
              n37 = local write "Current status"("Devices initialized") -> ()
              n38 = call <userlib>:"LVClass_WavefrontCorrector Get Current Position.vi"("WavefrontCorrector in"=w246, "error in (no error)"=w247) -> ("WavefrontCorrector out"=w231:refnum<class "WavefrontCorrector.lvclass">, "Wavefront Corrector Position"=→"Initial Positions":T14, "error out"=w229:errorcluster)  [unwired: 11 in]
              n39 = Increment(x=w227) -> (x+1=w226:i32)
            }
          }
        }
      }
    }
    n40 = local read "Exit"() -> (w57:bool)
    n41 = Or(x=w57, y="Init") -> (x .or. y?=w55:bool)
  }
  n42 = call <userlib>:"LVClass_HasoEngine ctor from file.vi"("HasoEngine in"=refnum<class "HasoEngine.lvclass"> refnum, "Configuration file path"="Haso configuration file") -> ("HasoEngine out"=w13:refnum<class "HasoEngine.lvclass">, "error out"=w14:errorcluster)  [unwired: 12 in]
  n43 = call <userlib>:"LVClass_HasoEngine Set Preferences.vi"("HasoEngine in"=w13, "Slopes_HasoEngine_Setup"=T10 {"Start sub-aperture"={"X"=16, "Y"=16}, "Pupil average"=1.0}, "error in (no error)"=w14) -> ("HasoEngine out"=w10:refnum<class "HasoEngine.lvclass">)  [unwired: 11 in, 1 out]
  n44 = while {
    shift-right: [w296] -> w46
    shift-left: w25 -> [w298]
    shift-right: [w294] -> w45
    shift-left: w38 -> [w295]
    shift-right: [w288] -> w44
    shift-left: w36 -> [w293]
    shift-right: [w287] -> w43
    shift-left: w35 -> [w292]
    shift-right: [w286] -> w42
    shift-left: w34 -> [w291]
    shift-right: [w285] -> w41
    shift-left: w33 -> [w290]
    shift-right: [w284] -> _
    shift-left: w39 -> [w289]
    shift-right: [w283] -> w40
    shift-left: w37 -> [w283]
    tunnel: w25 -> [w282]
    tunnel: w24 -> [w281]
    tunnel: w16 -> [w270]
    shift-right: [w278] -> w9
    shift-left: refnum<class "HasoSlopes.lvclass"> refnum ("HasoSlopes in") -> [w277]
    shift-right: [w276] -> w4
    shift-left: w10 -> [w279]
    shift-right: [w273] -> w5
    shift-left: refnum<class "Phase.lvclass"> refnum ("Phase in") -> [w275]
    shift-right: [w272] -> w3
    shift-left: refnum<class "Pupil.lvclass"> refnum ("Pupil in") -> [w274]
    tunnel: [w270] -> w2
    shift-right: [w269] -> w1
    shift-left: w17 -> [w271]
    stop <- w297 stop-if-true
    n45 = event shown="[6] \"Start HASO\": Mouse Up" {
      selector: _ -> [_ _ _ _ _ _ _ _ _ _ _ _ _]
      dyn-events: _ -> [_ _ _ _ _ _ _ _ _ _ _ _ _]
      timeout: 100 -> [_ _ _ _ _ _ _ _ _ _ _ _ _]
      tunnel: w298 -> [w314 w452 w455 w468 _ w515 w531 w549 w577 w668 w1191 _ w1731]
      tunnel: [w300 _ _ _ _ _ _ _ w578 w669 w1192 "Exit" TRUE ("Exit")] -> w297
      tunnel: [w301 w450 w455 w468 w486 w510 w529 w555 w576 w667 w1190 w1715 w1736] -> w296
      tunnel: w295 -> [w319 w451 w456 w469 w488 w514 w532 w556 w572 w656 w1179 w1716 w1738]
      tunnel: [w318 w449 w456 w469 w488 w511 w530 w557 w572 w656 w1179 w1714 w1737] -> w294
      tunnel: w293 -> [w322 w442 w463 w476 w490 w504 w527 w551 w588 w663 w1186 w1710 w1732]
      tunnel: w292 -> [w321 w443 w464 w477 w491 w505 w526 w552 w587 w662 w1185 w1711 w1733]
      tunnel: w291 -> [w320 w444 w465 w478 w492 w506 w525 w553 w586 w661 w1184 w1712 w1734]
      tunnel: w290 -> [w315 w445 w466 w479 w493 w507 w524 w554 w585 w660 w1183 w1713 w1735]
      tunnel: w289 -> [w311 w441 w462 w475 w489 w503 _ _ w573 w665 w1188 _ _]
      tunnel: [w317 w442 w463 w476 w490 w504 w527 w551 w588 w663 w1186 w1710 w1732] -> w288
      tunnel: [w316 w443 w464 w477 w491 w505 w526 w552 w587 w662 w1185 w1711 w1733] -> w287
      tunnel: [w313 w444 w465 w478 w492 w506 w525 w553 w586 w661 w1184 w1712 w1734] -> w286
      tunnel: [w312 w445 w466 w479 w493 w507 w524 w554 w585 w660 w1183 w1713 w1735] -> w285
      tunnel: [w311 w441 w462 w475 w489 w503 TRUE FALSE w573 w665 w1188 FALSE FALSE] -> w284
      tunnel: w282 -> [_ _ _ _ w485 _ _ _ _ _ _ _ _]
      tunnel: w281 -> [_ _ _ _ _ _ _ _ _ _ _ w1708 _]
      tunnel: w277 -> [w310 w439 w460 w473 w483 w497 w522 w547 w569 w658 w1181 w1706 w1728]
      tunnel: w279 -> [w309 w438 w459 w472 w482 w496 w521 w546 w568 w657 w1180 w1705 w1727]
      tunnel: [w308 w439 w460 w473 w483 w497 w522 w547 w569 w655 w1178 w1706 w1728] -> w278
      tunnel: [w307 w438 w459 w472 w482 w496 w521 w546 w568 w657 w1180 w1705 w1727] -> w276
      tunnel: w275 -> [w306 w440 w461 w474 w484 w498 w523 w548 w570 w659 w1182 w1707 w1729]
      tunnel: w274 -> [w305 w437 w458 w471 w481 w495 w520 w545 w567 w653 w1176 w1704 w1726]
      tunnel: [w304 w440 w461 w474 w484 w498 w523 w548 w570 w654 w1177 w1707 w1729] -> w273
      tunnel: [w303 w437 w458 w471 w481 w495 w520 w545 w567 w652 w1175 w1704 w1726] -> w272
      tunnel: w271 -> [w302 w436 w457 w470 w480 w494 w519 w544 w575 w666 w1189 w1703 w1725]
      tunnel: [w302 w436 w457 w470 w480 w494 w519 w544 w571 w664 w1187 w1703 w1725] -> w269
      event Timeout {
        n46 = event-data() -> ()  [unwired: 1 in, 2 out]
        n47 = case shown="True" w311 {
          tunnel: [w327 w348] -> w301
          tunnel: w322 -> [w332 w351]
          tunnel: [w332 w351] -> w317
          tunnel: [w328 w347] -> w316
          tunnel: w320 -> [w331 w350]
          tunnel: w315 -> [w330 w349]
          tunnel: [w331 w350] -> w313
          tunnel: [w330 w349] -> w312
          tunnel: w321 -> [w328 w347]
          tunnel: w319 -> [w329 w345]
          tunnel: [w329 w346] -> w318
          tunnel: w314 -> [w327 w344]
          tunnel: w310 -> [w325 w343]
          tunnel: w309 -> [w324 w342]
          tunnel: [w325 w341] -> w308
          tunnel: [w324 w340] -> w307
          tunnel: w306 -> [w326 w339]
          tunnel: w305 -> [w323 w338]
          tunnel: [w326 w337] -> w304
          tunnel: [w323 w336] -> w303
          frame False {
          }
          frame True {
            # "Acqure Wavefront Images"
            n48 = local read "HASO ready"() -> (w333:bool)
            n49 = And(x="Live Wavefront", y=w333) -> (x .and. y?=w335:bool)
            n50 = case shown="True" w335 {
              tunnel: w351 -> [_ w381]
              tunnel: w350 -> [_ w380]
              tunnel: w349 -> [_ w379]
              tunnel: [w352 w376] -> w348
              tunnel: w347 -> [_ w373]
              tunnel: [w357 w372] -> w346
              tunnel: w345 -> [w357 w371]
              tunnel: w344 -> [w352 w369]
              tunnel: w343 -> [w355 w367]
              tunnel: w342 -> [w354 w366]
              tunnel: [w355 w365] -> w341
              tunnel: [w354 w364] -> w340
              tunnel: w339 -> [w356 w363]
              tunnel: w338 -> [w353 w362]
              tunnel: [w356 w361] -> w337
              tunnel: [w353 w360] -> w336
              frame False {
              }
              frame True {
                n51 = property on="nb_images (set)" class="DigNum (strict)"() -> ("Value"=w382:u32)  [unwired: 2 in, 2 out]
                n52 = case shown="2, Default" w382 {
                  tunnel: [w433 w435] -> w383
                  tunnel: w373 -> [w432 _]
                  tunnel: w381 -> [w433 _]
                  tunnel: [w432 w434] -> w378
                  tunnel: w380 -> [_ w435]
                  tunnel: w379 -> [_ w434]
                  frame 2, Default {
                  }
                  frame 1 {
                  }
                }
                n53 = while {
                  tunnel: w371 -> [w431]
                  tunnel: [w430] -> w370
                  tunnel: w369 -> [w428]
                  tunnel: [w427] -> w368
                  stop <- w429 stop-if-true
                  n54 = call <userlib>:"LVClass_Camera asynchroneImageReady.vi"("Camera in"=w431, "error in (no error)"=w428) -> ("Camera out"=w430:refnum<class "Camera.lvclass">, "ready"=w429:bool, "error out"=w427:errorcluster)  [unwired: 11 in]
                }
                n55 = call <userlib>:"LVClass_Camera get image.vi"("Camera in"=w370, "Image"=w383, "Image RAW"=w378, "remove_background"=FALSE, "error in (no error)"=w368) -> ("Camera out"=w372:refnum<class "Camera.lvclass">, "Image (dup)"=w377:refnum<class "Image.lvclass">, "error out"=w374:errorcluster)  [unwired: 7 in, 1 out]
                n56 = case shown="No Error" w374 {
                  selector: w374 -> [w424 w425]
                  tunnel: w377 -> [w421 w426]
                  tunnel: [w419 w426] -> w359
                  tunnel: [w418 w425] -> w358
                  frame No Error {
                    # "get image"
                    n57 = call <userlib>:"LVClass_Image get image data.vi"("Image in"=w421, "error in (no error)"=w424) -> ("Image out"=w423:refnum<class "Image.lvclass">, "Image data out"=w417:u32[][], "error out"=w422:errorcluster)  [unwired: 11 in]
                    n58 = call <userlib>:"LVClass_Image get image information.vi"("Image in"=w423, "error in (no error)"=w422) -> ("Image out"=w419:refnum<class "Image.lvclass">, "Acquisition information"=→"Acquisition information":T5, "error out"=w418:errorcluster)  [unwired: 11 in]
                    n59 = local write "HASO intensity"(w417) -> ()
                  }
                  frame Error {
                  }
                }
                n60 = case shown="No Error" w358 {
                  selector: w358 -> [w404 w416]
                  tunnel: [w410 w416] -> w376
                  tunnel: w359 -> [w403 _]
                  tunnel: [w408 w412] -> w360
                  tunnel: [w407 w415] -> w361
                  tunnel: w367 -> [w400 w414]
                  tunnel: w366 -> [w399 w413]
                  tunnel: [w388 w414] -> w365
                  tunnel: [w398 w413] -> w364
                  tunnel: w363 -> [w396 w415]
                  tunnel: w362 -> [w394 w412]
                  frame No Error {
                    # "phaseout"
                    n61 = call "image2slopes.vi"("error in (no error)"=w404, "Image in"=w403, "HasoEngine in"=w399, "HasoSlopes in"=w400) -> ("error out"=w397:errorcluster, "HasoEngine out"=w398:refnum<class "HasoEngine.lvclass">, "HasoSlopes out"=w390:refnum<class "HasoSlopes.lvclass">)  [unwired: 4 in, 1 out]
                    n62 = local read "Filter"() -> (w393:u8[])
                    n63 = call "slopes2phase.vi"("TypePhase"=WavefrontReconstructionMode."Modal_Zernike", "Number of coefficients"=u8 32, "error in (no error)"=w397, "Filter"=w393, "HasoSlopes in"=w390, "Phase in"=w396) -> ("error out"=w387:errorcluster, "HasoSlopes out"=w389:refnum<class "HasoSlopes.lvclass">, "Phase out"=w395:refnum<class "Phase.lvclass">)  [unwired: 3 in]
                    n64 = local read "idxType"() -> (w384:enum16{"Wyant", "ANSI"})
                    n65 = call "slopes2zern.vi"("HasoSlopes in"=w389, "error in (no error)"=w387, "idxType"=w384) -> ("HasoSlopes out"=w388:refnum<class "HasoSlopes.lvclass">, "Zernike Coefficients"=w385:dbl[], "error out"=w386:errorcluster)  [unwired: 3 in, 2 out]
                    n66 = call <userlib>:"LVClass_Pupil ctor from HasoSlopes.vi"("Pupil in"=w394, "HasoSlopes.lvclass"=w390, "error in (no error)"=w386) -> ("Pupil out"=w405:refnum<class "Pupil.lvclass">, "error out"=w406:errorcluster)  [unwired: 11 in]
                    n67 = call <userlib>:"LVClasse_Phase GetStatisticDatas.vi"("Phase in"=w395, "error in (no error)"=w406) -> ("Phase out"=w411:refnum<class "Phase.lvclass">, "StatisticsData"=w391:T2, "error out"=w409:errorcluster)  [unwired: 11 in]
                    n68 = local write "Phase statistics"(w391) -> ()
                    n69 = call <userlib>:"LVClasse_Phase Get Data.vi"("Phase in"=w411, "Pupil"=w405, "error in (no error)"=w409) -> ("Phase out"=w407:refnum<class "Phase.lvclass">, "data"=w392:sgl[][], "Pupil (dup)"=w408:refnum<class "Pupil.lvclass">, "error out"=w410:errorcluster)  [unwired: 9 in]
                    n70 = local write "Zernike Measured"(w385) -> ()
                    n71 = local write "Phase values"(w392) -> ()
                  }
                  frame Error {
                  }
                }
              }
            }
          }
        }
        "Current error" <- w301
        n72 = Unbundle By Name(w301) -> ("status"=w300:bool)
      }
      event "nb_images (set)": Value Change {
        # "SET IMAGE NUMBER"
        n73 = event-data() -> ("NewVal"=w453:u32)  [unwired: 1 in]
        n74 = call <userlib>:"LVClass_Camera set nbImagesToSum.vi"("Camera in"=w451, "nb_image"=w453, "error in (no error)"=w452) -> ("Camera out"=w448:refnum<class "Camera.lvclass">, "error out"=w447:errorcluster)  [unwired: 11 in]
        n75 = call <userlib>:"LVClass_Camera get nbImagesToSum.vi"("Camera in"=w448, "error in (no error)"=w447) -> ("Camera out"=w449:refnum<class "Camera.lvclass">, "nb_image"=→"nb_images (get)":u32, "error out"=w450:errorcluster)  [unwired: 11 in]
      }
      event "Coef Min": Value Change {
        # "Set coeff display scale: min"
        n76 = event-data() -> ()  [unwired: 1 in, 1 out]
        n77 = local read "Coef Min"() -> (w454:dbl)
        n78 = property on="Zernike Measured" class="WFGraph (strict)"("YScale.Minimum"=w454) -> ()  [unwired: 2 in, 2 out]
      }
      event "Coef Max": Value Change {
        # "Set coeff display scale: min"
        n79 = event-data() -> ()  [unwired: 1 in, 1 out]
        n80 = local read "Coef Max"() -> (w467:dbl)
        n81 = property on="Zernike Measured" class="WFGraph (strict)"("YScale.Maximum"=w467) -> ()  [unwired: 2 in, 2 out]
      }
      event "Reset error": Mouse Up {
        n82 = event-data() -> ()  [unwired: 1 in, 8 out]
        n83 = Select(t=w485, s=w485, f=errorcluster {"status"=FALSE, "code"=0, "source"=""} ("error out")) -> (s? t:f=w486:errorcluster)
      }
      event "exposure_duration_s (set)": Value Change {
        # "CHANGE EXPOSURE DURATION"
        n84 = event-data() -> ()  [unwired: 1 in, 1 out]
        n85 = Multiply(x=1000000.0, y="exposure_duration_s (set)") -> (x*y=w501:dbl)
        n86 = To Unsigned Long Integer(number=w501) -> (unsigned 32bit integer=w500:u32)
        n87 = call <userlib>:"LVClass_Camera set Parameter Int.vi"("Camera in"=w514, "parameter_name"="exposure_duration_us", "value"=w500, "error in (no error)"=w515) -> ("Camera out"=w513:refnum<class "Camera.lvclass">, "error out"=w512:errorcluster)  [unwired: 10 in]
        n88 = call <userlib>:"LVClass_Camera get Parameter Int.vi"("Camera in"=w513, "parameter_name"="exposure_duration_us", "error in (no error)"=w512) -> ("Camera out"=w511:refnum<class "Camera.lvclass">, "value"=→"exposure_duration_us (get)":i32, "error out"=w510:errorcluster)  [unwired: 10 in]
      }
      event "Start HASO": Mouse Up {
        # "Start acquisition in SYNCRHONOUS mode\n\nonly one acquisition mode is available :\nLast image"
        n89 = event-data() -> ()  [unwired: 1 in, 8 out]
        n90 = flat-sequence {
          tunnel: w532 -> [w538]
          tunnel: w531 -> [w537]
          tunnel: [w536] -> w518
          tunnel: [w535] -> w517
          tunnel: [w540] -> w529
          tunnel: [w541] -> w530
          tunnel: w518 -> [w541]
          tunnel: w517 -> [w540]
          frame #0 {
            n91 = call <userlib>:"LVClass_Camera start acquisition.vi"("Camera in"=w538, "synchronisation_mode"=enum16{"synchronous", "asynchronous"}."asynchronous", "acquisition_mode"=enum16{"last_image", "new_image"}."last_image", "error in (no error)"=w537) -> ("Camera out"=w536:refnum<class "Camera.lvclass">, "error out"=w535:errorcluster)  [unwired: 10 in]
          }
          frame #1 {
            n92 = local write "HASO ready"(TRUE) -> ()
          }
        }
      }
      event "Stop HASO": Mouse Up {
        n93 = event-data() -> ()  [unwired: 1 in, 8 out]
        n94 = flat-sequence {
          tunnel: w556 -> [w560]
          tunnel: w549 -> [w558]
          tunnel: [w561] -> w543
          tunnel: [w559] -> w542
          tunnel: [w563] -> w555
          tunnel: [w564] -> w557
          tunnel: w543 -> [w564]
          tunnel: w542 -> [w563]
          frame #0 {
            n95 = call <userlib>:"LVClass_Camera stop acquisition.vi"("Camera in"=w560, "error in (no error)"=w558) -> ("Camera out"=w561:refnum<class "Camera.lvclass">, "error out"=w559:errorcluster)  [unwired: 12 in]
          }
          frame #1 {
            n96 = local write "HASO ready"(FALSE) -> ()
          }
        }
      }
      event "Update DM": Mouse Up {
        n97 = event-data() -> ()  [unwired: 1 in, 8 out]
        n98 = local read "Initial offset"() -> (w574:bool)
        n99 = case shown="True" w574 {
          tunnel: [w589 w594] -> w579
          frame False {
            n100 = Initialize Array(0.0, 52) -> (w589:dbl[])
          }
          frame True {
            n101 = local read "Offset command file"() -> (w593:path)
            n102 = call-poly <vilib>:"Read From Spreadsheet File.vi"("format (%.3f)"="%.8f", "file path (dialog if empty)"=w593) -> ("first row"=w594:dbl[])  [unwired: 5 in, 4 out]
          }
        }
        n103 = local read "Additional Command"() -> (w584:bool)
        n104 = case shown="True" w584 {
          tunnel: [w596 w602] -> w580
          tunnel: [w595 w601] -> w581
          tunnel: w577 -> [w595 w600]
          frame False {
            n105 = Initialize Array(0.0, 52) -> (w596:dbl[])
          }
          frame True {
            n106 = local read "Input type"() -> (w599:T4)
            n107 = case shown="\"Zero Input\"" w599 {
              tunnel: w600 -> [w603 w608 w622 w631]
              tunnel: [w604 w609 w620 w633] -> w602
              tunnel: [w603 w608 w619 w630] -> w601
              frame "Zero Input" {
                n108 = Initialize Array(0.0, 52) -> (w604:dbl[])
              }
              frame "Command File" {
                n109 = local read "Additional file"() -> (w607:path)
                n110 = call-poly <vilib>:"Read From Spreadsheet File.vi"("format (%.3f)"="%.8f", "file path (dialog if empty)"=w607) -> ("first row"=w609:dbl[])  [unwired: 5 in, 4 out]
              }
              frame "Zernike Coef", Default {
                n111 = local read "Zern index in"() -> (w611:i32[])
                n112 = local read "Zern coef in"() -> (w612:sgl[])
                n113 = local read "idxType"() -> (w618:enum16{"Wyant", "ANSI"})
                n114 = local read "Initial haso file"() -> (w616:path)
                n115 = local read "Haso configuration file"() -> (w617:path)
                n116 = local read "interaction matrix file"() -> (w615:path)
                n117 = call "zern2command.vi"("Haso configuration file"=w617, "idxType"=w618, "interaction matrix file"=w615, "error in (no error)"=w622, "Zern coef in"=w612, "Zern index in"=w611, "Initial haso file"=w616) -> ("error out"=w621:errorcluster, "Offset Positions"=w620:sgl[], "Zern pupil out"=w623:refnum<class "Pupil.lvclass">, "ModalCoef out"=w624:refnum<class "ModalCoef.lvclass">)  [unwired: 1 in]
                n118 = call <userlib>:"LVClass_ModalCoef GetData.vi"("ModalCoef in"=w624, "Pupil.lvclass"=w623, "error in (no error)"=w621) -> ("ModalCoef out"=w628:refnum<class "ModalCoef.lvclass">, "coef"=w614:sgl[], "index"=w613:u32[], "Pupil.lvclass (dup)"=w627:refnum<class "Pupil.lvclass">, "error out"=w626:errorcluster)  [unwired: 8 in]
                n119 = local write "Zern index out"(w613) -> ()
                n120 = call <userlib>:"LVClass_Pupil dtor.vi"("Pupil in"=w627, "error in (no error)"=w626) -> ("error out"=w625:errorcluster)  [unwired: 12 in, 1 out]
                n121 = local write "Zern coef out"(w614) -> ()
                n122 = call <userlib>:"LVClass_ModalCoef dtor.vi"("ModalCoef in"=w628, "error in (no error)"=w625) -> ("error out"=w619:errorcluster)  [unwired: 12 in, 1 out]
              }
              frame "Zernike File" {
                w636 = 1
                n123 = local read "interaction matrix file"() -> (w640:path)
                n124 = local read "Initial haso file"() -> (w638:path)
                n125 = local read "Haso configuration file"() -> (w639:path)
                n126 = local read "Additional file"() -> (w649:path)
                n127 = call-poly <vilib>:"Ramp Pattern.vi"("start"=w636, "end"=32, "delta"=w636) -> ("Ramp Pattern"=w637:dbl[])  [unwired: 6 in, 2 out]
                n128 = To Long Integer(number=w637) -> (32bit integer=w634:i32[])
                n129 = local read "idxType"() -> (w629:enum16{"Wyant", "ANSI"})
                n130 = call-poly <vilib>:"Read From Spreadsheet File.vi"("format (%.3f)"="%.8f", "file path (dialog if empty)"=w649) -> ("first row"=w641:dbl[])  [unwired: 5 in, 4 out]
                n131 = call "zern2command.vi"("Haso configuration file"=w639, "idxType"=w629, "interaction matrix file"=w640, "Zern coef in"=w641, "Zern index in"=w634, "Initial haso file"=w638) -> ("error out"=w642:errorcluster, "Offset Positions"=w633:sgl[], "Zern pupil out"=w643:refnum<class "Pupil.lvclass">, "ModalCoef out"=w644:refnum<class "ModalCoef.lvclass">)  [unwired: 2 in]
                n132 = call <userlib>:"LVClass_ModalCoef GetData.vi"("ModalCoef in"=w644, "Pupil.lvclass"=w643, "error in (no error)"=w642) -> ("ModalCoef out"=w648:refnum<class "ModalCoef.lvclass">, "Pupil.lvclass (dup)"=w647:refnum<class "Pupil.lvclass">, "error out"=w646:errorcluster)  [unwired: 8 in, 2 out]
                n133 = call <userlib>:"LVClass_Pupil dtor.vi"("Pupil in"=w647, "error in (no error)"=w646) -> ("error out"=w645:errorcluster)  [unwired: 12 in, 1 out]
                n134 = call <userlib>:"LVClass_ModalCoef dtor.vi"("ModalCoef in"=w648, "error in (no error)"=w645) -> ("error out"=w632:errorcluster)  [unwired: 12 in, 1 out]
                n135 = Merge Errors(w632, w631) -> (w630:errorcluster)
              }
            }
          }
        }
        n136 = local write "Initial Positions"(w579) -> ()
        n137 = Add(x=w580, y=w579) -> (x+y=w565:dbl[])
        n138 = call <userlib>:"LVClass_WavefrontCorrector Move to Absolute Position.vi"("WavefrontCorrector in"=w575, "Absolute Positions"=w565, "error in (no error)"=w581) -> ("WavefrontCorrector out"=w582:refnum<class "WavefrontCorrector.lvclass">, "error out"=w583:errorcluster)  [unwired: 11 in]
        n139 = call <userlib>:"LVClass_WavefrontCorrector Get Current Position.vi"("WavefrontCorrector in"=w582, "error in (no error)"=w583) -> ("WavefrontCorrector out"=w571:refnum<class "WavefrontCorrector.lvclass">, "Wavefront Corrector Position"=w566:T14, "error out"=w576:errorcluster)  [unwired: 11 in]
        n140 = local write "Final Positions"(w565) -> ()
        n141 = local write "DM Actuator Values"(w566) -> ()
        n142 = Unbundle By Name(w576) -> ("status"=w578:bool)
      }
      event "Record Response": Mouse Up {
        n143 = event-data() -> ()  [unwired: 1 in, 8 out]
        n144 = local read "Net Rp"() -> (w651:bool)
        n145 = stacked-sequence {
          seq-local: [_ _ _ w990 _] -> [_ _ _ _ w1012]
          seq-local: [_ _ w853 _ _] -> [_ _ _ w989 _]
          seq-local: [_ w694 _ _ _] -> [_ _ w854 _ _]
          seq-local: [_ _ w852 _ _] -> [_ _ _ _ w1008]
          tunnel: [_ _ _ _ w1011] -> w669
          tunnel: w668 -> [_ w706 _ _ _]
          tunnel: [_ _ _ _ w1010] -> w667
          tunnel: w666 -> [_ w705 _ w991 _]
          tunnel: [_ w703 _ _ _] -> w664
          tunnel: w663 -> [_ _ w866 _ w1020]
          tunnel: w662 -> [_ _ w865 _ w1019]
          tunnel: w661 -> [_ _ w864 _ w1018]
          tunnel: w660 -> [_ _ w863 _ w1017]
          tunnel: w659 -> [_ _ w862 _ w1016]
          tunnel: w658 -> [_ _ w861 _ _]
          tunnel: w657 -> [_ _ w860 _ w1015]
          tunnel: w653 -> [_ _ w859 _ w1014]
          tunnel: w656 -> [_ _ w858 _ w1013]
          tunnel: [_ _ _ _ w1007] -> w655
          tunnel: [_ _ w856 _ _] -> w654
          tunnel: [_ _ w855 _ _] -> w652
          tunnel: w651 -> [_ _ _ w988 w1009]
          frame #0 {
            # "Create output folder path"
            n146 = Get Date/Time In Seconds() -> (seconds since 1Jan1904=w681:timestamp)
            n147 = local read "Folder Name"() -> (w673:string)
            n148 = Format Date/Time String(time format string (%c)="%Y%m%d", seconds (now)=w681) -> (date/time string=w680:string)  [unwired: 1 in]
            n149 = local read "Main Path"() -> (w674:path)
            n150 = local read "Subfolder"() -> (w672:string)
            n151 = Concatenate Strings(w680, "_", w673) -> (w679:string)
            n152 = Build Path(base path=w674, name or relative path=w679) -> (appended path=w677:path)
            n153 = call <vilib>:"Check if File or Folder Exists.vi"("path"=w677) -> ("file or folder exists?"=w683:bool)  [unwired: 8 in, 2 out]
            n154 = local write "Current status"("Check single response") -> ()
            n155 = Build Path(base path=w677, name or relative path=w672) -> (appended path=w671:path)
            n156 = case shown="False" w683 {
              tunnel: w677 -> [w693 _]
              frame False {
                n157 = Create Folder(path (use dialog)=w693) -> ()  [unwired: 2 in, 3 out]
              }
              frame True {
              }
            }
            n158 = call <vilib>:"Check if File or Folder Exists.vi"("path"=w671) -> ("error out"=w678:errorcluster, "file or folder exists?"=w682:bool)  [unwired: 8 in, 1 out]
            n159 = case shown="True" w682 {
              tunnel: w671 -> [w686 w691]
              tunnel: w678 -> [w685 w692]
              tunnel: [w684 w687] -> _
              frame False {
                n160 = Create Folder(path (use dialog)=w686, error in=w685) -> (error out=w684:errorcluster)  [unwired: 1 in, 2 out]
              }
              frame True {
                n161 = Delete(path (use dialog)=w691, entire hierarchy (F)=TRUE, error in=w692) -> (deleted path=w689:path, error out=w688:errorcluster)  [unwired: 2 in, 1 out]
                n162 = Create Folder(path (use dialog)=w689, error in=w688) -> (error out=w687:errorcluster)  [unwired: 1 in, 2 out]
              }
            }
            n163 = local write "Output path"(w671) -> ()
          }
          frame #1 {
            # "Apply command to DM"
            n164 = local read "Initial offset"() -> (w704:bool)
            n165 = case shown="True" w704 {
              tunnel: [w790 w795] -> w695
              frame False {
                n166 = Initialize Array(0.0, 52) -> (w790:dbl[])
              }
              frame True {
                n167 = local read "Offset command file"() -> (w794:path)
                n168 = call-poly <vilib>:"Read From Spreadsheet File.vi"("format (%.3f)"="%.8f", "file path (dialog if empty)"=w794) -> ("first row"=w795:dbl[])  [unwired: 5 in, 4 out]
              }
            }
            n169 = local read "Additional Command"() -> (w710:bool)
            n170 = case shown="True" w710 {
              tunnel: [w797 w803] -> w696
              tunnel: [w796 w802] -> w707
              tunnel: w706 -> [w796 w801]
              frame False {
                n171 = Initialize Array(0.0, 52) -> (w797:dbl[])
              }
              frame True {
                n172 = local read "Input type"() -> (w800:T4)
                n173 = case shown="\"Zernike Coef\", Default" w800 {
                  tunnel: w801 -> [w804 w809 w823 w832]
                  tunnel: [w805 w810 w821 w834] -> w803
                  tunnel: [w804 w809 w820 w831] -> w802
                  frame "Zero Input" {
                    n174 = Initialize Array(0.0, 52) -> (w805:dbl[])
                  }
                  frame "Command File" {
                    n175 = local read "Additional file"() -> (w808:path)
                    n176 = call-poly <vilib>:"Read From Spreadsheet File.vi"("format (%.3f)"="%.8f", "file path (dialog if empty)"=w808) -> ("first row"=w810:dbl[])  [unwired: 5 in, 4 out]
                  }
                  frame "Zernike Coef", Default {
                    n177 = local read "Zern index in"() -> (w812:i32[])
                    n178 = local read "Zern coef in"() -> (w813:sgl[])
                    n179 = local read "idxType"() -> (w819:enum16{"Wyant", "ANSI"})
                    n180 = local read "Initial haso file"() -> (w817:path)
                    n181 = local read "Haso configuration file"() -> (w818:path)
                    n182 = local read "interaction matrix file"() -> (w816:path)
                    n183 = call "zern2command.vi"("Haso configuration file"=w818, "idxType"=w819, "interaction matrix file"=w816, "error in (no error)"=w823, "Zern coef in"=w813, "Zern index in"=w812, "Initial haso file"=w817) -> ("error out"=w822:errorcluster, "Offset Positions"=w821:sgl[], "Zern pupil out"=w824:refnum<class "Pupil.lvclass">, "ModalCoef out"=w825:refnum<class "ModalCoef.lvclass">)  [unwired: 1 in]
                    n184 = call <userlib>:"LVClass_ModalCoef GetData.vi"("ModalCoef in"=w825, "Pupil.lvclass"=w824, "error in (no error)"=w822) -> ("ModalCoef out"=w829:refnum<class "ModalCoef.lvclass">, "coef"=w815:sgl[], "index"=w814:u32[], "Pupil.lvclass (dup)"=w828:refnum<class "Pupil.lvclass">, "error out"=w827:errorcluster)  [unwired: 8 in]
                    n185 = local write "Zern index out"(w814) -> ()
                    n186 = call <userlib>:"LVClass_Pupil dtor.vi"("Pupil in"=w828, "error in (no error)"=w827) -> ("error out"=w826:errorcluster)  [unwired: 12 in, 1 out]
                    n187 = local write "Zern coef out"(w815) -> ()
                    n188 = call <userlib>:"LVClass_ModalCoef dtor.vi"("ModalCoef in"=w829, "error in (no error)"=w826) -> ("error out"=w820:errorcluster)  [unwired: 12 in, 1 out]
                  }
                  frame "Zernike File" {
                    w837 = 1
                    n189 = local read "interaction matrix file"() -> (w841:path)
                    n190 = local read "Initial haso file"() -> (w839:path)
                    n191 = local read "Haso configuration file"() -> (w840:path)
                    n192 = local read "Additional file"() -> (w850:path)
                    n193 = call-poly <vilib>:"Ramp Pattern.vi"("start"=w837, "end"=32, "delta"=w837) -> ("Ramp Pattern"=w838:dbl[])  [unwired: 6 in, 2 out]
                    n194 = To Long Integer(number=w838) -> (32bit integer=w835:i32[])
                    n195 = local read "idxType"() -> (w830:enum16{"Wyant", "ANSI"})
                    n196 = call-poly <vilib>:"Read From Spreadsheet File.vi"("format (%.3f)"="%.8f", "file path (dialog if empty)"=w850) -> ("first row"=w842:dbl[])  [unwired: 5 in, 4 out]
                    n197 = call "zern2command.vi"("Haso configuration file"=w840, "idxType"=w830, "interaction matrix file"=w841, "Zern coef in"=w842, "Zern index in"=w835, "Initial haso file"=w839) -> ("error out"=w843:errorcluster, "Offset Positions"=w834:sgl[], "Zern pupil out"=w844:refnum<class "Pupil.lvclass">, "ModalCoef out"=w845:refnum<class "ModalCoef.lvclass">)  [unwired: 2 in]
                    n198 = call <userlib>:"LVClass_ModalCoef GetData.vi"("ModalCoef in"=w845, "Pupil.lvclass"=w844, "error in (no error)"=w843) -> ("ModalCoef out"=w849:refnum<class "ModalCoef.lvclass">, "Pupil.lvclass (dup)"=w848:refnum<class "Pupil.lvclass">, "error out"=w847:errorcluster)  [unwired: 8 in, 2 out]
                    n199 = call <userlib>:"LVClass_Pupil dtor.vi"("Pupil in"=w848, "error in (no error)"=w847) -> ("error out"=w846:errorcluster)  [unwired: 12 in, 1 out]
                    n200 = call <userlib>:"LVClass_ModalCoef dtor.vi"("ModalCoef in"=w849, "error in (no error)"=w846) -> ("error out"=w833:errorcluster)  [unwired: 12 in, 1 out]
                    n201 = Merge Errors(w833, w832) -> (w831:errorcluster)
                  }
                }
              }
            }
            n202 = local read "File Base Name"() -> (w697:string)
            n203 = local read "Output path"() -> (w701:path)
            n204 = local read "Input type"() -> (w698:T4)
            n205 = local read "Save File"() -> (w702:bool)
            n206 = local write "Initial Positions"(w695) -> ()
            n207 = Add(x=w696, y=w695) -> (x+y=w699:dbl[])
            n208 = call <userlib>:"LVClass_WavefrontCorrector Move to Absolute Position.vi"("WavefrontCorrector in"=w705, "Absolute Positions"=w699, "error in (no error)"=w707) -> ("WavefrontCorrector out"=w708:refnum<class "WavefrontCorrector.lvclass">, "error out"=w709:errorcluster)  [unwired: 11 in]
            n209 = call <userlib>:"LVClass_WavefrontCorrector Get Current Position.vi"("WavefrontCorrector in"=w708, "error in (no error)"=w709) -> ("WavefrontCorrector out"=w703:refnum<class "WavefrontCorrector.lvclass">, "Wavefront Corrector Position"=w700:T14, "error out"=w694:errorcluster)  [unwired: 11 in]
            n210 = case shown="True" w702 {
              tunnel: w701 -> [_ w717]
              tunnel: w697 -> [_ w716]
              tunnel: w695 -> [_ w715]
              tunnel: w696 -> [_ w714]
              tunnel: w699 -> [_ w713]
              tunnel: w698 -> [_ w712]
              tunnel: w700 -> [_ w711]
              frame False {
              }
              frame True {
                n211 = stacked-sequence {
                  tunnel: w717 -> [w722 w731 w740 w749 w756 w768 w780]
                  tunnel: w716 -> [w720 w729 w738 w747 w755 w767 w779]
                  tunnel: w715 -> [w718 _ _ _ _ _ _]
                  tunnel: w714 -> [_ w727 _ _ _ _ _]
                  tunnel: w713 -> [_ _ w736 _ _ _ _]
                  tunnel: w712 -> [_ _ _ _ w754 w766 w778]
                  tunnel: w711 -> [_ _ _ w745 _ _ _]
                  frame #0 {
                    n212 = Concatenate Strings(w720, "_cmdOffset", ".dat") -> (w723:string)
                    n213 = Build Path(base path=w722, name or relative path=w723) -> (appended path=w724:path)
                    n214 = Array To Spreadsheet String(array=w718, 3:"%f") -> (spreadsheet string=w725:string)  [unwired: 1 in]
                    n215 = Write to Text File(file (use dialog)=w724, text=w725) -> ()  [unwired: 2 in, 3 out]
                  }
                  frame #1 {
                    n216 = Concatenate Strings(w729, "_cmdAdd", ".dat") -> (w732:string)
                    n217 = Build Path(base path=w731, name or relative path=w732) -> (appended path=w733:path)
                    n218 = Array To Spreadsheet String(array=w727, 3:"%f") -> (spreadsheet string=w734:string)  [unwired: 1 in]
                    n219 = Write to Text File(file (use dialog)=w733, text=w734) -> ()  [unwired: 2 in, 3 out]
                  }
                  frame #2 {
                    n220 = Concatenate Strings(w738, "_cmdFinal", ".dat") -> (w741:string)
                    n221 = Build Path(base path=w740, name or relative path=w741) -> (appended path=w742:path)
                    n222 = Array To Spreadsheet String(array=w736, 3:"%f") -> (spreadsheet string=w743:string)  [unwired: 1 in]
                    n223 = Write to Text File(file (use dialog)=w742, text=w743) -> ()  [unwired: 2 in, 3 out]
                  }
                  frame #3 {
                    n224 = Concatenate Strings(w747, "_cmdFinalMirror", ".dat") -> (w750:string)
                    n225 = Build Path(base path=w749, name or relative path=w750) -> (appended path=w751:path)
                    n226 = Array To Spreadsheet String(array=w745, 3:"%f") -> (spreadsheet string=w752:string)  [unwired: 1 in]
                    n227 = Write to Text File(file (use dialog)=w751, text=w752) -> ()  [unwired: 2 in, 3 out]
                  }
                  frame #4 {
                    n228 = case shown="\"Zernike Coef\", Default" w754 {
                      tunnel: w756 -> [_ w761]
                      tunnel: w755 -> [_ w759]
                      frame "Zero Input" {
                      }
                      frame "Zernike Coef", Default {
                        n229 = local read "Zern coef in"() -> (w757:sgl[])
                        n230 = Concatenate Strings(w759, "_zernCoef", ".txt") -> (w762:string)
                        n231 = Build Path(base path=w761, name or relative path=w762) -> (appended path=w763:path)
                        n232 = Array To Spreadsheet String(array=w757, 3:"%f") -> (spreadsheet string=w764:string)  [unwired: 1 in]
                        n233 = Write to Text File(file (use dialog)=w763, text=w764) -> ()  [unwired: 2 in, 3 out]
                      }
                    }
                  }
                  frame #5 {
                    n234 = case shown="\"Zernike Coef\", Default" w766 {
                      tunnel: w768 -> [_ w773]
                      tunnel: w767 -> [_ w771]
                      frame "Zero Input" {
                      }
                      frame "Zernike Coef", Default {
                        n235 = local read "Zern index in"() -> (w769:i32[])
                        n236 = Concatenate Strings(w771, "_zernIdx", ".txt") -> (w774:string)
                        n237 = Build Path(base path=w773, name or relative path=w774) -> (appended path=w775:path)
                        n238 = Array To Spreadsheet String(array=w769, 3:"%d") -> (spreadsheet string=w776:string)  [unwired: 1 in]
                        n239 = Write to Text File(file (use dialog)=w775, text=w776) -> ()  [unwired: 2 in, 3 out]
                      }
                    }
                  }
                  frame #6 {
                    n240 = case shown="\"Zernike Coef\", Default" w778 {
                      tunnel: w780 -> [_ w785]
                      tunnel: w779 -> [_ w783]
                      frame "Zero Input" {
                      }
                      frame "Zernike Coef", Default {
                        n241 = Concatenate Strings(w783, "_zernCoefWyant", ".txt") -> (w786:string)
                        n242 = local read "Zern coef out"() -> (w781:sgl[])
                        n243 = Build Path(base path=w785, name or relative path=w786) -> (appended path=w787:path)
                        n244 = Array To Spreadsheet String(array=w781, 3:"%f") -> (spreadsheet string=w788:string)  [unwired: 1 in]
                        n245 = Write to Text File(file (use dialog)=w787, text=w788) -> ()  [unwired: 2 in, 3 out]
                      }
                    }
                  }
                }
              }
            }
            n246 = local write "Final Positions"(w699) -> ()
            n247 = local write "DM Actuator Values"(w700) -> ()
          }
          frame #2 {
            n248 = local read "HASO ready"() -> (w857:bool)
            n249 = case shown="True" w857 {
              tunnel: w866 -> [_ w893]
              tunnel: w864 -> [_ w892]
              tunnel: w863 -> [_ w891]
              tunnel: [w867 w888] -> w853
              tunnel: w865 -> [_ w886]
              tunnel: [w872 w885] -> _
              tunnel: w858 -> [w872 w884]
              tunnel: w854 -> [w867 w883]
              tunnel: w861 -> [w870 w882]
              tunnel: w860 -> [w869 w881]
              tunnel: [w870 w880] -> w852
              tunnel: [w869 w879] -> _
              tunnel: w862 -> [w871 w878]
              tunnel: w859 -> [w868 w877]
              tunnel: [w871 w876] -> w856
              tunnel: [w868 w875] -> w855
              frame False {
              }
              frame True {
                n250 = property on="nb_images (set)" class="DigNum (strict)"() -> ("Value"=w894:u32)  [unwired: 2 in, 2 out]
                n251 = case shown="2, Default" w894 {
                  tunnel: [w985 w987] -> w895
                  tunnel: w886 -> [w984 _]
                  tunnel: w893 -> [w985 _]
                  tunnel: [w984 w986] -> w890
                  tunnel: w892 -> [_ w987]
                  tunnel: w891 -> [_ w986]
                  frame 2, Default {
                  }
                  frame 1 {
                  }
                }
                n252 = stacked-sequence {
                  tunnel: w895 -> [_ w913]
                  tunnel: w890 -> [_ w912]
                  tunnel: [_ w911] -> w889
                  tunnel: [_ w909] -> w887
                  tunnel: [_ w908] -> w885
                  tunnel: w884 -> [_ w905]
                  tunnel: w883 -> [_ w904]
                  frame #0 {
                    # "Delay until MD gets stable"
                    n253 = local read "exposure_duration_s (set)"() -> (w898:dbl)
                    n254 = local read "nb_images (set)"() -> (w897:u32)
                    n255 = Multiply(x=w898, y=w897) -> (x*y=w896:dbl)
                    n256 = Add(x=w896, y=1.0) -> (x+y=w899:dbl)
                    n257 = Multiply(x=w899, y=1000.0) -> (x*y=w903:dbl)
                    n258 = To Unsigned Long Integer(number=w903) -> (unsigned 32bit integer=w902:u32)
                    n259 = Wait (ms)(milliseconds to wait=w902) -> ()  [unwired: 1 out]
                  }
                  frame #1 {
                    n260 = while {
                      tunnel: w905 -> [w918]
                      tunnel: [w917] -> w907
                      tunnel: w904 -> [w915]
                      tunnel: [w914] -> w906
                      stop <- w916 stop-if-true
                      n261 = call <userlib>:"LVClass_Camera asynchroneImageReady.vi"("Camera in"=w918, "error in (no error)"=w915) -> ("Camera out"=w917:refnum<class "Camera.lvclass">, "ready"=w916:bool, "error out"=w914:errorcluster)  [unwired: 11 in]
                    }
                    n262 = call <userlib>:"LVClass_Camera get image.vi"("Camera in"=w907, "Image"=w913, "Image RAW"=w912, "remove_background"=FALSE, "error in (no error)"=w906) -> ("Camera out"=w908:refnum<class "Camera.lvclass">, "Image (dup)"=w911:refnum<class "Image.lvclass">, "error out"=w909:errorcluster)  [unwired: 7 in, 1 out]
                  }
                }
                n263 = case shown="No Error" w887 {
                  selector: w887 -> [w981 w982]
                  tunnel: w889 -> [w978 w983]
                  tunnel: [w977 w983] -> w874
                  tunnel: [w976 w982] -> w873
                  frame No Error {
                    # "get image"
                    n264 = call <userlib>:"LVClass_Image get image data.vi"("Image in"=w978, "error in (no error)"=w981) -> ("Image out"=w980:refnum<class "Image.lvclass">, "Image data out"=w975:u32[][], "error out"=w979:errorcluster)  [unwired: 11 in]
                    n265 = call <userlib>:"LVClass_Image get image information.vi"("Image in"=w980, "error in (no error)"=w979) -> ("Image out"=w977:refnum<class "Image.lvclass">, "error out"=w976:errorcluster)  [unwired: 11 in, 1 out]
                    n266 = local write "HASO intensity"(w975) -> ()
                  }
                  frame Error {
                  }
                }
                n267 = case shown="No Error" w873 {
                  selector: w873 -> [w942 w974]
                  tunnel: [w948 w974] -> w888
                  tunnel: w874 -> [w941 _]
                  tunnel: [w946 w970] -> w875
                  tunnel: [w945 w973] -> w876
                  tunnel: w882 -> [w938 w972]
                  tunnel: w881 -> [w937 w971]
                  tunnel: [w925 w972] -> w880
                  tunnel: [w936 w971] -> w879
                  tunnel: w878 -> [w934 w973]
                  tunnel: w877 -> [w932 w970]
                  frame No Error {
                    # "phaseout"
                    n268 = local read "File Base Name"() -> (w923:string)
                    n269 = local read "Save File"() -> (w924:bool)
                    n270 = local read "Output path"() -> (w922:path)
                    n271 = call "image2slopes.vi"("error in (no error)"=w942, "Image in"=w941, "HasoEngine in"=w937, "HasoSlopes in"=w938) -> ("error out"=w935:errorcluster, "HasoEngine out"=w936:refnum<class "HasoEngine.lvclass">, "HasoSlopes out"=w919:refnum<class "HasoSlopes.lvclass">)  [unwired: 4 in, 1 out]
                    n272 = local read "Filter"() -> (w931:u8[])
                    n273 = call "slopes2phase.vi"("TypePhase"=WavefrontReconstructionMode."Modal_Zernike", "Number of coefficients"=u8 32, "error in (no error)"=w935, "Filter"=w931, "HasoSlopes in"=w919, "Phase in"=w934) -> ("error out"=w927:errorcluster, "HasoSlopes out"=w928:refnum<class "HasoSlopes.lvclass">, "Phase out"=w933:refnum<class "Phase.lvclass">)  [unwired: 3 in]
                    n274 = local read "idxType"() -> (w921:enum16{"Wyant", "ANSI"})
                    n275 = call "slopes2zern.vi"("HasoSlopes in"=w928, "error in (no error)"=w927, "idxType"=w921) -> ("HasoSlopes out"=w925:refnum<class "HasoSlopes.lvclass">, "Zernike Coefficients"=w920:dbl[], "error out"=w926:errorcluster)  [unwired: 3 in, 2 out]
                    n276 = call <userlib>:"LVClass_Pupil ctor from HasoSlopes.vi"("Pupil in"=w932, "HasoSlopes.lvclass"=w919, "error in (no error)"=w926) -> ("Pupil out"=w943:refnum<class "Pupil.lvclass">, "error out"=w944:errorcluster)  [unwired: 11 in]
                    n277 = case shown="True" w924 {
                      tunnel: w923 -> [_ w953]
                      tunnel: w922 -> [_ w952]
                      tunnel: w920 -> [_ w951]
                      tunnel: w919 -> [_ w950]
                      frame False {
                      }
                      frame True {
                        n278 = stacked-sequence {
                          tunnel: w953 -> [w957 w963]
                          tunnel: w952 -> [w956 w962]
                          tunnel: w951 -> [_ w961]
                          tunnel: w950 -> [w954 _]
                          frame #0 {
                            n279 = Concatenate Strings(w957, "_slopesMeas", ".has") -> (w960:string)
                            n280 = Build Path(base path=w956, name or relative path=w960) -> (appended path=w955:path)
                            n281 = call <userlib>:"LVClass_HasoSlopes Save.vi"("HasoSlopes in"=w954, "path"=w955) -> ()  [unwired: 12 in, 2 out]
                          }
                          frame #1 {
                            n282 = Concatenate Strings(w963, "_zernCoefMeas", ".txt") -> (w966:string)
                            n283 = Build Path(base path=w962, name or relative path=w966) -> (appended path=w967:path)
                            n284 = Array To Spreadsheet String(array=w961, 3:"%f") -> (spreadsheet string=w968:string)  [unwired: 1 in]
                            n285 = Write to Text File(file (use dialog)=w967, text=w968) -> ()  [unwired: 2 in, 3 out]
                          }
                        }
                      }
                    }
                    n286 = call <userlib>:"LVClasse_Phase GetStatisticDatas.vi"("Phase in"=w933, "error in (no error)"=w944) -> ("Phase out"=w949:refnum<class "Phase.lvclass">, "StatisticsData"=w929:T2, "error out"=w947:errorcluster)  [unwired: 11 in]
                    n287 = local write "Phase statistics"(w929) -> ()
                    n288 = call <userlib>:"LVClasse_Phase Get Data.vi"("Phase in"=w949, "Pupil"=w943, "error in (no error)"=w947) -> ("Phase out"=w945:refnum<class "Phase.lvclass">, "data"=w930:sgl[][], "Pupil (dup)"=w946:refnum<class "Pupil.lvclass">, "error out"=w948:errorcluster)  [unwired: 9 in]
                    n289 = local write "Zernike Measured"(w920) -> ()
                    n290 = local write "Phase values"(w930) -> ()
                  }
                  frame Error {
                  }
                }
              }
            }
          }
          frame #3 {
            # "Apply offset to DM"
            n291 = case shown="True" w988 {
              tunnel: w991 -> [_ w998]
              tunnel: [w992 w994] -> w990
              tunnel: w989 -> [w992 w993]
              frame False {
              }
              frame True {
                n292 = local read "Initial offset"() -> (w997:bool)
                n293 = case shown="True" w997 {
                  tunnel: [w1001 w1006] -> w995
                  frame False {
                    n294 = Initialize Array(0.0, 52) -> (w1001:dbl[])
                  }
                  frame True {
                    n295 = local read "Offset command file"() -> (w1005:path)
                    n296 = call-poly <vilib>:"Read From Spreadsheet File.vi"("format (%.3f)"="%.8f", "file path (dialog if empty)"=w1005) -> ("first row"=w1006:dbl[])  [unwired: 5 in, 4 out]
                  }
                }
                n297 = local write "Initial Positions"(w995) -> ()
                n298 = call <userlib>:"LVClass_WavefrontCorrector Move to Absolute Position.vi"("WavefrontCorrector in"=w998, "Absolute Positions"=w995, "error in (no error)"=w993) -> ("WavefrontCorrector out"=w999:refnum<class "WavefrontCorrector.lvclass">, "error out"=w1000:errorcluster)  [unwired: 11 in]
                n299 = call <userlib>:"LVClass_WavefrontCorrector Get Current Position.vi"("WavefrontCorrector in"=w999, "error in (no error)"=w1000) -> ("Wavefront Corrector Position"=w996:T14, "error out"=w994:errorcluster)  [unwired: 11 in, 1 out]
                n300 = local write "Initial Positions"(w996) -> ()
              }
            }
          }
          frame #4 {
            n301 = case shown="True" w1009 {
              tunnel: w1020 -> [_ w1035]
              tunnel: w1019 -> [_ w1034]
              tunnel: w1018 -> [_ w1033]
              tunnel: w1017 -> [_ w1032]
              tunnel: w1016 -> [_ w1031]
              tunnel: w1008 -> [w1021 w1030]
              tunnel: w1015 -> [_ w1029]
              tunnel: w1014 -> [_ w1028]
              tunnel: w1013 -> [_ w1027]
              tunnel: w1012 -> [w1022 w1025]
              tunnel: [w1022 w1024] -> w1010
              tunnel: [w1021 w1023] -> w1007
              frame False {
              }
              frame True {
                n302 = local read "HASO ready"() -> (w1026:bool)
                n303 = case shown="True" w1026 {
                  tunnel: w1035 -> [_ w1064]
                  tunnel: w1033 -> [_ w1063]
                  tunnel: w1032 -> [_ w1062]
                  tunnel: [w1036 w1059] -> w1024
                  tunnel: w1034 -> [_ w1057]
                  tunnel: [w1041 w1056] -> _
                  tunnel: w1027 -> [w1041 w1055]
                  tunnel: w1025 -> [w1036 w1045]
                  tunnel: w1030 -> [w1039 w1042]
                  tunnel: w1029 -> [w1038 w1054]
                  tunnel: [w1039 w1044] -> w1023
                  tunnel: [w1038 w1053] -> _
                  tunnel: w1031 -> [w1040 w1052]
                  tunnel: w1028 -> [w1037 w1051]
                  tunnel: [w1040 w1050] -> _
                  tunnel: [w1037 w1049] -> _
                  frame False {
                  }
                  frame True {
                    n304 = property on="nb_images (set)" class="DigNum (strict)"() -> ("Value"=w1065:u32)  [unwired: 2 in, 2 out]
                    n305 = case shown="2, Default" w1065 {
                      tunnel: [w1168 w1170] -> w1066
                      tunnel: w1057 -> [w1167 _]
                      tunnel: w1064 -> [w1168 _]
                      tunnel: [w1167 w1169] -> w1061
                      tunnel: w1063 -> [_ w1170]
                      tunnel: w1062 -> [_ w1169]
                      frame 2, Default {
                      }
                      frame 1 {
                      }
                    }
                    n306 = stacked-sequence {
                      tunnel: w1066 -> [_ w1084]
                      tunnel: w1061 -> [_ w1083]
                      tunnel: [_ w1082] -> w1060
                      tunnel: [_ w1080] -> w1058
                      tunnel: [_ w1079] -> w1056
                      tunnel: w1055 -> [_ w1076]
                      tunnel: w1045 -> [_ w1075]
                      frame #0 {
                        # "Delay until MD gets stable"
                        n307 = local read "exposure_duration_s (set)"() -> (w1069:dbl)
                        n308 = local read "nb_images (set)"() -> (w1068:u32)
                        n309 = Multiply(x=w1069, y=w1068) -> (x*y=w1067:dbl)
                        n310 = Add(x=w1067, y=1.0) -> (x+y=w1070:dbl)
                        n311 = Multiply(x=w1070, y=1000.0) -> (x*y=w1074:dbl)
                        n312 = To Unsigned Long Integer(number=w1074) -> (unsigned 32bit integer=w1073:u32)
                        n313 = Wait (ms)(milliseconds to wait=w1073) -> ()  [unwired: 1 out]
                      }
                      frame #1 {
                        n314 = while {
                          tunnel: w1076 -> [w1089]
                          tunnel: [w1088] -> w1078
                          tunnel: w1075 -> [w1086]
                          tunnel: [w1085] -> w1077
                          stop <- w1087 stop-if-true
                          n315 = call <userlib>:"LVClass_Camera asynchroneImageReady.vi"("Camera in"=w1089, "error in (no error)"=w1086) -> ("Camera out"=w1088:refnum<class "Camera.lvclass">, "ready"=w1087:bool, "error out"=w1085:errorcluster)  [unwired: 11 in]
                        }
                        n316 = call <userlib>:"LVClass_Camera get image.vi"("Camera in"=w1078, "Image"=w1084, "Image RAW"=w1083, "remove_background"=FALSE, "error in (no error)"=w1077) -> ("Camera out"=w1079:refnum<class "Camera.lvclass">, "Image (dup)"=w1082:refnum<class "Image.lvclass">, "error out"=w1080:errorcluster)  [unwired: 7 in, 1 out]
                      }
                    }
                    n317 = case shown="No Error" w1058 {
                      selector: w1058 -> [w1164 w1165]
                      tunnel: w1060 -> [w1161 w1166]
                      tunnel: [w1160 w1166] -> w1048
                      tunnel: [w1159 w1165] -> w1047
                      frame No Error {
                        # "get image"
                        n318 = call <userlib>:"LVClass_Image get image data.vi"("Image in"=w1161, "error in (no error)"=w1164) -> ("Image out"=w1163:refnum<class "Image.lvclass">, "Image data out"=w1158:u32[][], "error out"=w1162:errorcluster)  [unwired: 11 in]
                        n319 = call <userlib>:"LVClass_Image get image information.vi"("Image in"=w1163, "error in (no error)"=w1162) -> ("Image out"=w1160:refnum<class "Image.lvclass">, "error out"=w1159:errorcluster)  [unwired: 11 in, 1 out]
                        n320 = local write "HASO intensity"(w1158) -> ()
                      }
                      frame Error {
                      }
                    }
                    n321 = case shown="No Error" w1047 {
                      selector: w1047 -> [w1116 w1157]
                      tunnel: [w1122 w1157] -> w1059
                      tunnel: w1048 -> [w1115 _]
                      tunnel: [w1120 w1154] -> w1049
                      tunnel: [w1119 w1156] -> w1050
                      tunnel: refnum<class "HasoSlopes.lvclass"> refnum ("HasoSlopes in") -> [w1112 w1153]
                      tunnel: w1054 -> [w1111 w1155]
                      tunnel: [w1110 w1155] -> w1053
                      tunnel: w1052 -> [w1109 w1156]
                      tunnel: w1051 -> [w1107 w1154]
                      tunnel: [w1092 w1152] -> w1044
                      tunnel: [w1090 w1153] -> w1043
                      tunnel: w1042 -> [w1091 w1152]
                      frame No Error {
                        # "phaseout"
                        n322 = local read "File Base Name"() -> (w1099:string)
                        n323 = local read "Save File"() -> (w1100:bool)
                        n324 = local read "Output path"() -> (w1098:path)
                        n325 = call "image2slopes.vi"("error in (no error)"=w1116, "Image in"=w1115, "HasoEngine in"=w1111, "HasoSlopes in"=w1112) -> ("error out"=w1094:errorcluster, "HasoEngine out"=w1110:refnum<class "HasoEngine.lvclass">, "HasoSlopes out"=w1090:refnum<class "HasoSlopes.lvclass">)  [unwired: 4 in, 1 out]
                        n326 = local read "Filter"() -> (w1106:u8[])
                        n327 = call <userlib>:"LVClass_HasoSlopes Apply Substractor.vi"("HasoSlopes in"=w1091, "HasoSlopes to substract"=w1090, "error in (no error)"=w1094) -> ("HasoSlopes out"=w1095:refnum<class "HasoSlopes.lvclass">, "error out"=w1093:errorcluster)  [unwired: 11 in]
                        n328 = call "slopes2phase.vi"("TypePhase"=WavefrontReconstructionMode."Modal_Zernike", "Number of coefficients"=u8 32, "error in (no error)"=w1093, "Filter"=w1106, "HasoSlopes in"=w1095, "Phase in"=w1109) -> ("error out"=w1102:errorcluster, "HasoSlopes out"=w1103:refnum<class "HasoSlopes.lvclass">, "Phase out"=w1108:refnum<class "Phase.lvclass">)  [unwired: 3 in]
                        n329 = local read "idxType"() -> (w1097:enum16{"Wyant", "ANSI"})
                        n330 = call "slopes2zern.vi"("HasoSlopes in"=w1103, "error in (no error)"=w1102, "idxType"=w1097) -> ("HasoSlopes out"=w1092:refnum<class "HasoSlopes.lvclass">, "Zernike Coefficients"=w1096:dbl[], "error out"=w1101:errorcluster)  [unwired: 3 in, 2 out]
                        n331 = call <userlib>:"LVClass_Pupil ctor from HasoSlopes.vi"("Pupil in"=w1107, "HasoSlopes.lvclass"=w1095, "error in (no error)"=w1101) -> ("Pupil out"=w1117:refnum<class "Pupil.lvclass">, "error out"=w1118:errorcluster)  [unwired: 11 in]
                        n332 = case shown="True" w1100 {
                          tunnel: w1099 -> [_ w1128]
                          tunnel: w1098 -> [_ w1127]
                          tunnel: w1096 -> [_ w1126]
                          tunnel: w1095 -> [_ w1124]
                          tunnel: w1090 -> [_ w1125]
                          frame False {
                          }
                          frame True {
                            n333 = stacked-sequence {
                              tunnel: w1128 -> [w1132 w1139 w1145]
                              tunnel: w1127 -> [w1131 w1138 w1144]
                              tunnel: w1126 -> [_ _ w1143]
                              tunnel: w1125 -> [w1129 _ _]
                              tunnel: w1124 -> [_ w1136 _]
                              frame #0 {
                                n334 = Concatenate Strings(w1132, "_slopesOffset", ".has") -> (w1135:string)
                                n335 = Build Path(base path=w1131, name or relative path=w1135) -> (appended path=w1130:path)
                                n336 = call <userlib>:"LVClass_HasoSlopes Save.vi"("HasoSlopes in"=w1129, "path"=w1130) -> ()  [unwired: 12 in, 2 out]
                              }
                              frame #1 {
                                n337 = Concatenate Strings(w1139, "_slopesNet", ".has") -> (w1142:string)
                                n338 = Build Path(base path=w1138, name or relative path=w1142) -> (appended path=w1137:path)
                                n339 = call <userlib>:"LVClass_HasoSlopes Save.vi"("HasoSlopes in"=w1136, "path"=w1137) -> ()  [unwired: 12 in, 2 out]
                              }
                              frame #2 {
                                n340 = Concatenate Strings(w1145, "_zernCoefNet", ".txt") -> (w1148:string)
                                n341 = Build Path(base path=w1144, name or relative path=w1148) -> (appended path=w1149:path)
                                n342 = Array To Spreadsheet String(array=w1143, 3:"%f") -> (spreadsheet string=w1150:string)  [unwired: 1 in]
                                n343 = Write to Text File(file (use dialog)=w1149, text=w1150) -> ()  [unwired: 2 in, 3 out]
                              }
                            }
                          }
                        }
                        n344 = call <userlib>:"LVClasse_Phase GetStatisticDatas.vi"("Phase in"=w1108, "error in (no error)"=w1118) -> ("Phase out"=w1123:refnum<class "Phase.lvclass">, "StatisticsData"=w1104:T2, "error out"=w1121:errorcluster)  [unwired: 11 in]
                        n345 = local write "Phase statistics"(w1104) -> ()
                        n346 = call <userlib>:"LVClasse_Phase Get Data.vi"("Phase in"=w1123, "Pupil"=w1117, "error in (no error)"=w1121) -> ("Phase out"=w1119:refnum<class "Phase.lvclass">, "data"=w1105:sgl[][], "Pupil (dup)"=w1120:refnum<class "Pupil.lvclass">, "error out"=w1122:errorcluster)  [unwired: 9 in]
                        n347 = local write "Zernike Measured"(w1096) -> ()
                        n348 = local write "Phase values"(w1105) -> ()
                      }
                      frame Error {
                      }
                    }
                    n349 = call <userlib>:"LVClass_HasoSlopes dtor.vi"("HasoSlopes in"=w1043) -> ()  [unwired: 13 in, 2 out]
                  }
                }
              }
            }
            n350 = Unbundle By Name(w1010) -> ("status"=w1011:bool)
          }
        }
      }
      event "Record Batch": Mouse Up {
        n351 = event-data() -> ()  [unwired: 1 in, 8 out]
        n352 = local read "Idx start"() -> (w1171:u32)
        n353 = local read "Idx end"() -> (w1172:u32)
        n354 = Subtract(x=w1172, y=w1171) -> (x-y=w1173:u32)
        n355 = Increment(x=w1173) -> (x+1=w1174:u32)
        n356 = for {
          N: w1174 -> [_]
          tunnel: [w1213] -> w1192
          tunnel: w1186 -> [w1208]
          tunnel: w1185 -> [w1207]
          tunnel: w1184 -> [w1206]
          tunnel: w1183 -> [w1205]
          tunnel: w1180 -> [w1202]
          tunnel: w1179 -> [w1201]
          shift-right: [w1211] -> w1190
          shift-left: w1191 -> [w1212]
          shift-right: [w1209] -> w1187
          shift-left: w1189 -> [w1210]
          shift-right: [w1199] -> w1177
          shift-left: w1182 -> [w1204]
          shift-right: [w1200] -> w1178
          shift-left: w1181 -> [w1203]
          shift-right: [w1197] -> w1175
          shift-left: w1176 -> [w1198]
          tunnel: w1171 -> [w1194]
          i -> [w1195]
          n357 = Add(x=w1194, y=w1195) -> (x+y=w1193:u32)
          n358 = local read "Net Rp"() -> (w1196:bool)
          n359 = stacked-sequence {
            seq-local: [_ _ _ w1522 _] -> [_ _ _ _ w1544]
            seq-local: [_ _ w1385 _ _] -> [_ _ _ w1521 _]
            seq-local: [_ w1257 _ _ _] -> [_ _ w1386 _ _]
            seq-local: [_ _ w1384 _ _] -> [_ _ _ _ w1540]
            tunnel: [_ _ _ _ w1543] -> w1213
            tunnel: w1212 -> [_ w1269 _ _ _]
            tunnel: [_ _ _ _ w1542] -> w1211
            tunnel: w1210 -> [_ w1268 _ w1523 _]
            tunnel: [_ w1266 _ _ _] -> w1209
            tunnel: w1208 -> [_ _ w1398 _ w1552]
            tunnel: w1207 -> [_ _ w1397 _ w1551]
            tunnel: w1206 -> [_ _ w1396 _ w1550]
            tunnel: w1205 -> [_ _ w1395 _ w1549]
            tunnel: w1204 -> [_ _ w1394 _ w1548]
            tunnel: w1203 -> [_ _ w1393 _ _]
            tunnel: w1202 -> [_ _ w1392 _ w1547]
            tunnel: w1198 -> [_ _ w1391 _ w1546]
            tunnel: w1201 -> [_ _ w1390 _ w1545]
            tunnel: [_ _ _ _ w1539] -> w1200
            tunnel: [_ _ w1388 _ _] -> w1199
            tunnel: [_ _ w1387 _ _] -> w1197
            tunnel: w1196 -> [_ _ _ w1520 w1541]
            tunnel: w1193 -> [w1215 w1256 _ _ _]
            frame #0 {
              # "Create output folder path"
              n360 = Get Date/Time In Seconds() -> (seconds since 1Jan1904=w1236:timestamp)
              n361 = local read "Folder Name"() -> (w1228:string)
              n362 = local read "idxType"() -> (w1219:enum16{"Wyant", "ANSI"})
              n363 = Number To Decimal String(number=w1215) -> (decimal integer string=w1216:string)  [unwired: 1 in]
              n364 = Format Date/Time String(time format string (%c)="%Y%m%d", seconds (now)=w1236) -> (date/time string=w1235:string)  [unwired: 1 in]
              n365 = local read "Main Path"() -> (w1229:path)
              n366 = case shown="\"ANSI\"" w1219 {
                tunnel: ["Wyant" "ANSI"] -> w1218
                frame "Wyant", Default {
                }
                frame "ANSI" {
                }
              }
              n367 = local read "Subfolder"() -> (w1227:string)
              n368 = Concatenate Strings(w1235, "_", w1228) -> (w1234:string)
              n369 = Build Path(base path=w1229, name or relative path=w1234) -> (appended path=w1232:path)
              n370 = call <vilib>:"Check if File or Folder Exists.vi"("path"=w1232) -> ("error out"=w1225:errorcluster, "file or folder exists?"=w1238:bool)  [unwired: 8 in, 1 out]
              n371 = Concatenate Strings(w1218, "_idx_", w1216) -> (w1214:string)
              n372 = Build Path(base path=w1232, name or relative path=w1227) -> (appended path=w1223:path)
              n373 = Build Path(base path=w1223, name or relative path=w1214) -> (appended path=w1220:path)
              n374 = local write "Current status"(w1214) -> ()
              n375 = case shown="False" w1238 {
                tunnel: w1232 -> [w1254 _]
                tunnel: w1225 -> [w1253 w1255]
                tunnel: [w1252 w1255] -> w1224
                frame False {
                  n376 = Create Folder(path (use dialog)=w1254, error in=w1253) -> (error out=w1252:errorcluster)  [unwired: 1 in, 2 out]
                }
                frame True {
                }
              }
              n377 = call <vilib>:"Check if File or Folder Exists.vi"("error in (no error)"=w1224, "path"=w1223) -> ("error out"=w1222:errorcluster, "file or folder exists?"=w1226:bool)  [unwired: 7 in, 1 out]
              n378 = case shown="True" w1226 {
                tunnel: w1223 -> [w1243 _]
                tunnel: w1222 -> [w1242 w1244]
                tunnel: [w1241 w1244] -> w1221
                frame False {
                  n379 = Create Folder(path (use dialog)=w1243, error in=w1242) -> (error out=w1241:errorcluster)  [unwired: 1 in, 2 out]
                }
                frame True {
                }
              }
              n380 = call <vilib>:"Check if File or Folder Exists.vi"("error in (no error)"=w1221, "path"=w1220) -> ("error out"=w1233:errorcluster, "file or folder exists?"=w1237:bool)  [unwired: 7 in, 1 out]
              n381 = case shown="False" w1237 {
                tunnel: w1220 -> [w1246 w1250]
                tunnel: w1233 -> [w1245 w1251]
                frame False {
                  n382 = Create Folder(path (use dialog)=w1246, error in=w1245) -> ()  [unwired: 1 in, 3 out]
                }
                frame True {
                  n383 = Delete(path (use dialog)=w1250, entire hierarchy (F)=TRUE, error in=w1251) -> (deleted path=w1248:path, error out=w1247:errorcluster)  [unwired: 2 in, 1 out]
                  n384 = Create Folder(path (use dialog)=w1248, error in=w1247) -> ()  [unwired: 1 in, 3 out]
                }
              }
              n385 = local write "Output path"(w1220) -> ()
            }
            frame #1 {
              # "Apply command to DM"
              n386 = local read "Initial offset"() -> (w1267:bool)
              n387 = case shown="True" w1267 {
                tunnel: [w1353 w1358] -> w1258
                frame False {
                  n388 = Initialize Array(0.0, 52) -> (w1353:dbl[])
                }
                frame True {
                  n389 = local read "Offset command file"() -> (w1357:path)
                  n390 = call-poly <vilib>:"Read From Spreadsheet File.vi"("format (%.3f)"="%.8f", "file path (dialog if empty)"=w1357) -> ("first row"=w1358:dbl[])  [unwired: 5 in, 4 out]
                }
              }
              n391 = local read "Additional Command"() -> (w1273:bool)
              n392 = case shown="True" w1273 {
                tunnel: [w1360 w1383] -> w1259
                tunnel: [w1359 w1382] -> w1270
                tunnel: w1269 -> [w1359 w1381]
                tunnel: w1256 -> [_ w1364]
                frame False {
                  n393 = Initialize Array(0.0, 52) -> (w1360:dbl[])
                }
                frame True {
                  w1365 = 1
                  n394 = local read "Coef value"() -> (w1367:dbl)
                  n395 = local read "Initial haso file"() -> (w1371:path)
                  n396 = Initialize Array(w1364, w1365) -> (w1363:u32[])
                  n397 = Initialize Array(w1367, w1365) -> (w1366:dbl[])
                  n398 = local read "Haso configuration file"() -> (w1372:path)
                  n399 = local read "interaction matrix file"() -> (w1370:path)
                  n400 = local read "idxType"() -> (w1373:enum16{"Wyant", "ANSI"})
                  n401 = call "zern2command.vi"("Haso configuration file"=w1372, "idxType"=w1373, "interaction matrix file"=w1370, "error in (no error)"=w1381, "Zern coef in"=w1366, "Zern index in"=w1363, "Initial haso file"=w1371) -> ("error out"=w1374:errorcluster, "Offset Positions"=w1383:sgl[], "Zern pupil out"=w1375:refnum<class "Pupil.lvclass">, "ModalCoef out"=w1376:refnum<class "ModalCoef.lvclass">)  [unwired: 1 in]
                  n402 = call <userlib>:"LVClass_ModalCoef GetData.vi"("ModalCoef in"=w1376, "Pupil.lvclass"=w1375, "error in (no error)"=w1374) -> ("ModalCoef out"=w1380:refnum<class "ModalCoef.lvclass">, "coef"=w1369:sgl[], "index"=w1368:u32[], "Pupil.lvclass (dup)"=w1379:refnum<class "Pupil.lvclass">, "error out"=w1378:errorcluster)  [unwired: 8 in]
                  n403 = local write "Zern index out"(w1368) -> ()
                  n404 = call <userlib>:"LVClass_Pupil dtor.vi"("Pupil in"=w1379, "error in (no error)"=w1378) -> ("error out"=w1377:errorcluster)  [unwired: 12 in, 1 out]
                  n405 = local write "Zern coef out"(w1369) -> ()
                  n406 = call <userlib>:"LVClass_ModalCoef dtor.vi"("ModalCoef in"=w1380, "error in (no error)"=w1377) -> ("error out"=w1382:errorcluster)  [unwired: 12 in, 1 out]
                }
              }
              n407 = local read "File Base Name"() -> (w1260:string)
              n408 = local read "Output path"() -> (w1264:path)
              n409 = local read "Input type"() -> (w1261:T4)
              n410 = local read "Save File"() -> (w1265:bool)
              n411 = local write "Initial Positions"(w1258) -> ()
              n412 = Add(x=w1259, y=w1258) -> (x+y=w1262:dbl[])
              n413 = call <userlib>:"LVClass_WavefrontCorrector Move to Absolute Position.vi"("WavefrontCorrector in"=w1268, "Absolute Positions"=w1262, "error in (no error)"=w1270) -> ("WavefrontCorrector out"=w1271:refnum<class "WavefrontCorrector.lvclass">, "error out"=w1272:errorcluster)  [unwired: 11 in]
              n414 = call <userlib>:"LVClass_WavefrontCorrector Get Current Position.vi"("WavefrontCorrector in"=w1271, "error in (no error)"=w1272) -> ("WavefrontCorrector out"=w1266:refnum<class "WavefrontCorrector.lvclass">, "Wavefront Corrector Position"=w1263:T14, "error out"=w1257:errorcluster)  [unwired: 11 in]
              n415 = case shown="True" w1265 {
                tunnel: w1264 -> [_ w1280]
                tunnel: w1260 -> [_ w1279]
                tunnel: w1258 -> [_ w1278]
                tunnel: w1259 -> [_ w1277]
                tunnel: w1262 -> [_ w1276]
                tunnel: w1261 -> [_ w1275]
                tunnel: w1263 -> [_ w1274]
                frame False {
                }
                frame True {
                  n416 = stacked-sequence {
                    tunnel: w1280 -> [w1285 w1294 w1303 w1312 w1319 w1331 w1343]
                    tunnel: w1279 -> [w1283 w1292 w1301 w1310 w1318 w1330 w1342]
                    tunnel: w1278 -> [w1281 _ _ _ _ _ _]
                    tunnel: w1277 -> [_ w1290 _ _ _ _ _]
                    tunnel: w1276 -> [_ _ w1299 _ _ _ _]
                    tunnel: w1275 -> [_ _ _ _ w1317 w1329 w1341]
                    tunnel: w1274 -> [_ _ _ w1308 _ _ _]
                    frame #0 {
                      n417 = Concatenate Strings(w1283, "_cmdOffset", ".dat") -> (w1286:string)
                      n418 = Build Path(base path=w1285, name or relative path=w1286) -> (appended path=w1287:path)
                      n419 = Array To Spreadsheet String(array=w1281, 3:"%f") -> (spreadsheet string=w1288:string)  [unwired: 1 in]
                      n420 = Write to Text File(file (use dialog)=w1287, text=w1288) -> ()  [unwired: 2 in, 3 out]
                    }
                    frame #1 {
                      n421 = Concatenate Strings(w1292, "_cmdAdd", ".dat") -> (w1295:string)
                      n422 = Build Path(base path=w1294, name or relative path=w1295) -> (appended path=w1296:path)
                      n423 = Array To Spreadsheet String(array=w1290, 3:"%f") -> (spreadsheet string=w1297:string)  [unwired: 1 in]
                      n424 = Write to Text File(file (use dialog)=w1296, text=w1297) -> ()  [unwired: 2 in, 3 out]
                    }
                    frame #2 {
                      n425 = Concatenate Strings(w1301, "_cmdFinal", ".dat") -> (w1304:string)
                      n426 = Build Path(base path=w1303, name or relative path=w1304) -> (appended path=w1305:path)
                      n427 = Array To Spreadsheet String(array=w1299, 3:"%f") -> (spreadsheet string=w1306:string)  [unwired: 1 in]
                      n428 = Write to Text File(file (use dialog)=w1305, text=w1306) -> ()  [unwired: 2 in, 3 out]
                    }
                    frame #3 {
                      n429 = Concatenate Strings(w1310, "_cmdFinalMirror", ".dat") -> (w1313:string)
                      n430 = Build Path(base path=w1312, name or relative path=w1313) -> (appended path=w1314:path)
                      n431 = Array To Spreadsheet String(array=w1308, 3:"%f") -> (spreadsheet string=w1315:string)  [unwired: 1 in]
                      n432 = Write to Text File(file (use dialog)=w1314, text=w1315) -> ()  [unwired: 2 in, 3 out]
                    }
                    frame #4 {
                      n433 = case shown="\"Zernike Coef\", Default" w1317 {
                        tunnel: w1319 -> [_ w1324]
                        tunnel: w1318 -> [_ w1322]
                        frame "Zero Input" {
                        }
                        frame "Zernike Coef", Default {
                          n434 = local read "Zern coef in"() -> (w1320:sgl[])
                          n435 = Concatenate Strings(w1322, "_zernCoef", ".txt") -> (w1325:string)
                          n436 = Build Path(base path=w1324, name or relative path=w1325) -> (appended path=w1326:path)
                          n437 = Array To Spreadsheet String(array=w1320, 3:"%f") -> (spreadsheet string=w1327:string)  [unwired: 1 in]
                          n438 = Write to Text File(file (use dialog)=w1326, text=w1327) -> ()  [unwired: 2 in, 3 out]
                        }
                      }
                    }
                    frame #5 {
                      n439 = case shown="\"Zernike Coef\", Default" w1329 {
                        tunnel: w1331 -> [_ w1336]
                        tunnel: w1330 -> [_ w1334]
                        frame "Zero Input" {
                        }
                        frame "Zernike Coef", Default {
                          n440 = local read "Zern index in"() -> (w1332:i32[])
                          n441 = Concatenate Strings(w1334, "_zernIdx", ".txt") -> (w1337:string)
                          n442 = Build Path(base path=w1336, name or relative path=w1337) -> (appended path=w1338:path)
                          n443 = Array To Spreadsheet String(array=w1332, 3:"%d") -> (spreadsheet string=w1339:string)  [unwired: 1 in]
                          n444 = Write to Text File(file (use dialog)=w1338, text=w1339) -> ()  [unwired: 2 in, 3 out]
                        }
                      }
                    }
                    frame #6 {
                      n445 = case shown="\"Zernike Coef\", Default" w1341 {
                        tunnel: w1343 -> [_ w1348]
                        tunnel: w1342 -> [_ w1346]
                        frame "Zero Input" {
                        }
                        frame "Zernike Coef", Default {
                          n446 = Concatenate Strings(w1346, "_zernCoefWyant", ".txt") -> (w1349:string)
                          n447 = local read "Zern coef out"() -> (w1344:sgl[])
                          n448 = Build Path(base path=w1348, name or relative path=w1349) -> (appended path=w1350:path)
                          n449 = Array To Spreadsheet String(array=w1344, 3:"%f") -> (spreadsheet string=w1351:string)  [unwired: 1 in]
                          n450 = Write to Text File(file (use dialog)=w1350, text=w1351) -> ()  [unwired: 2 in, 3 out]
                        }
                      }
                    }
                  }
                }
              }
              n451 = local write "Final Positions"(w1262) -> ()
              n452 = local write "DM Actuator Values"(w1263) -> ()
            }
            frame #2 {
              n453 = local read "HASO ready"() -> (w1389:bool)
              n454 = case shown="True" w1389 {
                tunnel: w1398 -> [_ w1425]
                tunnel: w1396 -> [_ w1424]
                tunnel: w1395 -> [_ w1423]
                tunnel: [w1399 w1420] -> w1385
                tunnel: w1397 -> [_ w1418]
                tunnel: [w1404 w1417] -> _
                tunnel: w1390 -> [w1404 w1416]
                tunnel: w1386 -> [w1399 w1415]
                tunnel: w1393 -> [w1402 w1414]
                tunnel: w1392 -> [w1401 w1413]
                tunnel: [w1402 w1412] -> w1384
                tunnel: [w1401 w1411] -> _
                tunnel: w1394 -> [w1403 w1410]
                tunnel: w1391 -> [w1400 w1409]
                tunnel: [w1403 w1408] -> w1388
                tunnel: [w1400 w1407] -> w1387
                frame False {
                }
                frame True {
                  n455 = property on="nb_images (set)" class="DigNum (strict)"() -> ("Value"=w1426:u32)  [unwired: 2 in, 2 out]
                  n456 = case shown="2, Default" w1426 {
                    tunnel: [w1517 w1519] -> w1427
                    tunnel: w1418 -> [w1516 _]
                    tunnel: w1425 -> [w1517 _]
                    tunnel: [w1516 w1518] -> w1422
                    tunnel: w1424 -> [_ w1519]
                    tunnel: w1423 -> [_ w1518]
                    frame 2, Default {
                    }
                    frame 1 {
                    }
                  }
                  n457 = stacked-sequence {
                    tunnel: w1427 -> [_ w1445]
                    tunnel: w1422 -> [_ w1444]
                    tunnel: [_ w1443] -> w1421
                    tunnel: [_ w1441] -> w1419
                    tunnel: [_ w1440] -> w1417
                    tunnel: w1416 -> [_ w1437]
                    tunnel: w1415 -> [_ w1436]
                    frame #0 {
                      # "Delay until MD gets stable"
                      n458 = local read "exposure_duration_s (set)"() -> (w1430:dbl)
                      n459 = local read "nb_images (set)"() -> (w1429:u32)
                      n460 = Multiply(x=w1430, y=w1429) -> (x*y=w1428:dbl)
                      n461 = Add(x=w1428, y=3.0) -> (x+y=w1431:dbl)
                      n462 = Multiply(x=w1431, y=1000.0) -> (x*y=w1435:dbl)
                      n463 = To Unsigned Long Integer(number=w1435) -> (unsigned 32bit integer=w1434:u32)
                      n464 = Wait (ms)(milliseconds to wait=w1434) -> ()  [unwired: 1 out]
                    }
                    frame #1 {
                      n465 = while {
                        tunnel: w1437 -> [w1450]
                        tunnel: [w1449] -> w1439
                        tunnel: w1436 -> [w1447]
                        tunnel: [w1446] -> w1438
                        stop <- w1448 stop-if-true
                        n466 = call <userlib>:"LVClass_Camera asynchroneImageReady.vi"("Camera in"=w1450, "error in (no error)"=w1447) -> ("Camera out"=w1449:refnum<class "Camera.lvclass">, "ready"=w1448:bool, "error out"=w1446:errorcluster)  [unwired: 11 in]
                      }
                      n467 = call <userlib>:"LVClass_Camera get image.vi"("Camera in"=w1439, "Image"=w1445, "Image RAW"=w1444, "remove_background"=FALSE, "error in (no error)"=w1438) -> ("Camera out"=w1440:refnum<class "Camera.lvclass">, "Image (dup)"=w1443:refnum<class "Image.lvclass">, "error out"=w1441:errorcluster)  [unwired: 7 in, 1 out]
                    }
                  }
                  n468 = case shown="No Error" w1419 {
                    selector: w1419 -> [w1513 w1514]
                    tunnel: w1421 -> [w1510 w1515]
                    tunnel: [w1509 w1515] -> w1406
                    tunnel: [w1508 w1514] -> w1405
                    frame No Error {
                      # "get image"
                      n469 = call <userlib>:"LVClass_Image get image data.vi"("Image in"=w1510, "error in (no error)"=w1513) -> ("Image out"=w1512:refnum<class "Image.lvclass">, "Image data out"=w1507:u32[][], "error out"=w1511:errorcluster)  [unwired: 11 in]
                      n470 = call <userlib>:"LVClass_Image get image information.vi"("Image in"=w1512, "error in (no error)"=w1511) -> ("Image out"=w1509:refnum<class "Image.lvclass">, "error out"=w1508:errorcluster)  [unwired: 11 in, 1 out]
                      n471 = local write "HASO intensity"(w1507) -> ()
                    }
                    frame Error {
                    }
                  }
                  n472 = case shown="No Error" w1405 {
                    selector: w1405 -> [w1474 w1506]
                    tunnel: [w1480 w1506] -> w1420
                    tunnel: w1406 -> [w1473 _]
                    tunnel: [w1478 w1502] -> w1407
                    tunnel: [w1477 w1505] -> w1408
                    tunnel: w1414 -> [w1470 w1504]
                    tunnel: w1413 -> [w1469 w1503]
                    tunnel: [w1457 w1504] -> w1412
                    tunnel: [w1468 w1503] -> w1411
                    tunnel: w1410 -> [w1466 w1505]
                    tunnel: w1409 -> [w1464 w1502]
                    frame No Error {
                      # "phaseout"
                      n473 = local read "File Base Name"() -> (w1455:string)
                      n474 = local read "Save File"() -> (w1456:bool)
                      n475 = local read "Output path"() -> (w1454:path)
                      n476 = call "image2slopes.vi"("error in (no error)"=w1474, "Image in"=w1473, "HasoEngine in"=w1469, "HasoSlopes in"=w1470) -> ("error out"=w1467:errorcluster, "HasoEngine out"=w1468:refnum<class "HasoEngine.lvclass">, "HasoSlopes out"=w1451:refnum<class "HasoSlopes.lvclass">)  [unwired: 4 in, 1 out]
                      n477 = local read "Filter"() -> (w1463:u8[])
                      n478 = call "slopes2phase.vi"("TypePhase"=WavefrontReconstructionMode."Modal_Zernike", "Number of coefficients"=u8 32, "error in (no error)"=w1467, "Filter"=w1463, "HasoSlopes in"=w1451, "Phase in"=w1466) -> ("error out"=w1459:errorcluster, "HasoSlopes out"=w1460:refnum<class "HasoSlopes.lvclass">, "Phase out"=w1465:refnum<class "Phase.lvclass">)  [unwired: 3 in]
                      n479 = local read "idxType"() -> (w1453:enum16{"Wyant", "ANSI"})
                      n480 = call "slopes2zern.vi"("HasoSlopes in"=w1460, "error in (no error)"=w1459, "idxType"=w1453) -> ("HasoSlopes out"=w1457:refnum<class "HasoSlopes.lvclass">, "Zernike Coefficients"=w1452:dbl[], "error out"=w1458:errorcluster)  [unwired: 3 in, 2 out]
                      n481 = call <userlib>:"LVClass_Pupil ctor from HasoSlopes.vi"("Pupil in"=w1464, "HasoSlopes.lvclass"=w1451, "error in (no error)"=w1458) -> ("Pupil out"=w1475:refnum<class "Pupil.lvclass">, "error out"=w1476:errorcluster)  [unwired: 11 in]
                      n482 = case shown="True" w1456 {
                        tunnel: w1455 -> [_ w1485]
                        tunnel: w1454 -> [_ w1484]
                        tunnel: w1452 -> [_ w1483]
                        tunnel: w1451 -> [_ w1482]
                        frame False {
                        }
                        frame True {
                          n483 = stacked-sequence {
                            tunnel: w1485 -> [w1489 w1495]
                            tunnel: w1484 -> [w1488 w1494]
                            tunnel: w1483 -> [_ w1493]
                            tunnel: w1482 -> [w1486 _]
                            frame #0 {
                              n484 = Concatenate Strings(w1489, "_slopesMeas", ".has") -> (w1492:string)
                              n485 = Build Path(base path=w1488, name or relative path=w1492) -> (appended path=w1487:path)
                              n486 = call <userlib>:"LVClass_HasoSlopes Save.vi"("HasoSlopes in"=w1486, "path"=w1487) -> ()  [unwired: 12 in, 2 out]
                            }
                            frame #1 {
                              n487 = Concatenate Strings(w1495, "_zernCoefMeas", ".txt") -> (w1498:string)
                              n488 = Build Path(base path=w1494, name or relative path=w1498) -> (appended path=w1499:path)
                              n489 = Array To Spreadsheet String(array=w1493, 3:"%f") -> (spreadsheet string=w1500:string)  [unwired: 1 in]
                              n490 = Write to Text File(file (use dialog)=w1499, text=w1500) -> ()  [unwired: 2 in, 3 out]
                            }
                          }
                        }
                      }
                      n491 = call <userlib>:"LVClasse_Phase GetStatisticDatas.vi"("Phase in"=w1465, "error in (no error)"=w1476) -> ("Phase out"=w1481:refnum<class "Phase.lvclass">, "StatisticsData"=w1461:T2, "error out"=w1479:errorcluster)  [unwired: 11 in]
                      n492 = local write "Phase statistics"(w1461) -> ()
                      n493 = call <userlib>:"LVClasse_Phase Get Data.vi"("Phase in"=w1481, "Pupil"=w1475, "error in (no error)"=w1479) -> ("Phase out"=w1477:refnum<class "Phase.lvclass">, "data"=w1462:sgl[][], "Pupil (dup)"=w1478:refnum<class "Pupil.lvclass">, "error out"=w1480:errorcluster)  [unwired: 9 in]
                      n494 = local write "Zernike Measured"(w1452) -> ()
                      n495 = local write "Phase values"(w1462) -> ()
                    }
                    frame Error {
                    }
                  }
                }
              }
            }
            frame #3 {
              # "Apply offset to DM"
              n496 = case shown="True" w1520 {
                tunnel: w1523 -> [_ w1530]
                tunnel: [w1524 w1526] -> w1522
                tunnel: w1521 -> [w1524 w1525]
                frame False {
                }
                frame True {
                  n497 = local read "Initial offset"() -> (w1529:bool)
                  n498 = case shown="True" w1529 {
                    tunnel: [w1533 w1538] -> w1527
                    frame False {
                      n499 = Initialize Array(0.0, 52) -> (w1533:dbl[])
                    }
                    frame True {
                      n500 = local read "Offset command file"() -> (w1537:path)
                      n501 = call-poly <vilib>:"Read From Spreadsheet File.vi"("format (%.3f)"="%.8f", "file path (dialog if empty)"=w1537) -> ("first row"=w1538:dbl[])  [unwired: 5 in, 4 out]
                    }
                  }
                  n502 = local write "Initial Positions"(w1527) -> ()
                  n503 = call <userlib>:"LVClass_WavefrontCorrector Move to Absolute Position.vi"("WavefrontCorrector in"=w1530, "Absolute Positions"=w1527, "error in (no error)"=w1525) -> ("WavefrontCorrector out"=w1531:refnum<class "WavefrontCorrector.lvclass">, "error out"=w1532:errorcluster)  [unwired: 11 in]
                  n504 = call <userlib>:"LVClass_WavefrontCorrector Get Current Position.vi"("WavefrontCorrector in"=w1531, "error in (no error)"=w1532) -> ("Wavefront Corrector Position"=w1528:T14, "error out"=w1526:errorcluster)  [unwired: 11 in, 1 out]
                  n505 = local write "Initial Positions"(w1528) -> ()
                }
              }
            }
            frame #4 {
              n506 = case shown="True" w1541 {
                tunnel: w1552 -> [_ w1567]
                tunnel: w1551 -> [_ w1566]
                tunnel: w1550 -> [_ w1565]
                tunnel: w1549 -> [_ w1564]
                tunnel: w1548 -> [_ w1563]
                tunnel: w1540 -> [w1553 w1562]
                tunnel: w1547 -> [_ w1561]
                tunnel: w1546 -> [_ w1560]
                tunnel: w1545 -> [_ w1559]
                tunnel: w1544 -> [w1554 w1557]
                tunnel: [w1554 w1556] -> w1542
                tunnel: [w1553 w1555] -> w1539
                frame False {
                }
                frame True {
                  n507 = local read "HASO ready"() -> (w1558:bool)
                  n508 = case shown="True" w1558 {
                    tunnel: w1567 -> [_ w1596]
                    tunnel: w1565 -> [_ w1595]
                    tunnel: w1564 -> [_ w1594]
                    tunnel: [w1568 w1591] -> w1556
                    tunnel: w1566 -> [_ w1589]
                    tunnel: [w1573 w1588] -> _
                    tunnel: w1559 -> [w1573 w1587]
                    tunnel: w1557 -> [w1568 w1577]
                    tunnel: w1562 -> [w1571 w1574]
                    tunnel: w1561 -> [w1570 w1586]
                    tunnel: [w1571 w1576] -> w1555
                    tunnel: [w1570 w1585] -> _
                    tunnel: w1563 -> [w1572 w1584]
                    tunnel: w1560 -> [w1569 w1583]
                    tunnel: [w1572 w1582] -> _
                    tunnel: [w1569 w1581] -> _
                    frame False {
                    }
                    frame True {
                      n509 = property on="nb_images (set)" class="DigNum (strict)"() -> ("Value"=w1597:u32)  [unwired: 2 in, 2 out]
                      n510 = case shown="2, Default" w1597 {
                        tunnel: [w1700 w1702] -> w1598
                        tunnel: w1589 -> [w1699 _]
                        tunnel: w1596 -> [w1700 _]
                        tunnel: [w1699 w1701] -> w1593
                        tunnel: w1595 -> [_ w1702]
                        tunnel: w1594 -> [_ w1701]
                        frame 2, Default {
                        }
                        frame 1 {
                        }
                      }
                      n511 = stacked-sequence {
                        tunnel: w1598 -> [_ w1616]
                        tunnel: w1593 -> [_ w1615]
                        tunnel: [_ w1614] -> w1592
                        tunnel: [_ w1612] -> w1590
                        tunnel: [_ w1611] -> w1588
                        tunnel: w1587 -> [_ w1608]
                        tunnel: w1577 -> [_ w1607]
                        frame #0 {
                          # "Delay until MD gets stable"
                          n512 = local read "exposure_duration_s (set)"() -> (w1601:dbl)
                          n513 = local read "nb_images (set)"() -> (w1600:u32)
                          n514 = Multiply(x=w1601, y=w1600) -> (x*y=w1599:dbl)
                          n515 = Add(x=w1599, y=3.0) -> (x+y=w1602:dbl)
                          n516 = Multiply(x=w1602, y=1000.0) -> (x*y=w1606:dbl)
                          n517 = To Unsigned Long Integer(number=w1606) -> (unsigned 32bit integer=w1605:u32)
                          n518 = Wait (ms)(milliseconds to wait=w1605) -> ()  [unwired: 1 out]
                        }
                        frame #1 {
                          n519 = while {
                            tunnel: w1608 -> [w1621]
                            tunnel: [w1620] -> w1610
                            tunnel: w1607 -> [w1618]
                            tunnel: [w1617] -> w1609
                            stop <- w1619 stop-if-true
                            n520 = call <userlib>:"LVClass_Camera asynchroneImageReady.vi"("Camera in"=w1621, "error in (no error)"=w1618) -> ("Camera out"=w1620:refnum<class "Camera.lvclass">, "ready"=w1619:bool, "error out"=w1617:errorcluster)  [unwired: 11 in]
                          }
                          n521 = call <userlib>:"LVClass_Camera get image.vi"("Camera in"=w1610, "Image"=w1616, "Image RAW"=w1615, "remove_background"=FALSE, "error in (no error)"=w1609) -> ("Camera out"=w1611:refnum<class "Camera.lvclass">, "Image (dup)"=w1614:refnum<class "Image.lvclass">, "error out"=w1612:errorcluster)  [unwired: 7 in, 1 out]
                        }
                      }
                      n522 = case shown="No Error" w1590 {
                        selector: w1590 -> [w1696 w1697]
                        tunnel: w1592 -> [w1693 w1698]
                        tunnel: [w1692 w1698] -> w1580
                        tunnel: [w1691 w1697] -> w1579
                        frame No Error {
                          # "get image"
                          n523 = call <userlib>:"LVClass_Image get image data.vi"("Image in"=w1693, "error in (no error)"=w1696) -> ("Image out"=w1695:refnum<class "Image.lvclass">, "Image data out"=w1690:u32[][], "error out"=w1694:errorcluster)  [unwired: 11 in]
                          n524 = call <userlib>:"LVClass_Image get image information.vi"("Image in"=w1695, "error in (no error)"=w1694) -> ("Image out"=w1692:refnum<class "Image.lvclass">, "error out"=w1691:errorcluster)  [unwired: 11 in, 1 out]
                          n525 = local write "HASO intensity"(w1690) -> ()
                        }
                        frame Error {
                        }
                      }
                      n526 = case shown="No Error" w1579 {
                        selector: w1579 -> [w1648 w1689]
                        tunnel: [w1654 w1689] -> w1591
                        tunnel: w1580 -> [w1647 _]
                        tunnel: [w1652 w1686] -> w1581
                        tunnel: [w1651 w1688] -> w1582
                        tunnel: refnum<class "HasoSlopes.lvclass"> refnum ("HasoSlopes in") -> [w1644 w1685]
                        tunnel: w1586 -> [w1643 w1687]
                        tunnel: [w1642 w1687] -> w1585
                        tunnel: w1584 -> [w1641 w1688]
                        tunnel: w1583 -> [w1639 w1686]
                        tunnel: [w1624 w1684] -> w1576
                        tunnel: [w1622 w1685] -> w1575
                        tunnel: w1574 -> [w1623 w1684]
                        frame No Error {
                          # "phaseout"
                          n527 = local read "File Base Name"() -> (w1631:string)
                          n528 = local read "Save File"() -> (w1632:bool)
                          n529 = local read "Output path"() -> (w1630:path)
                          n530 = call "image2slopes.vi"("error in (no error)"=w1648, "Image in"=w1647, "HasoEngine in"=w1643, "HasoSlopes in"=w1644) -> ("error out"=w1626:errorcluster, "HasoEngine out"=w1642:refnum<class "HasoEngine.lvclass">, "HasoSlopes out"=w1622:refnum<class "HasoSlopes.lvclass">)  [unwired: 4 in, 1 out]
                          n531 = local read "Filter"() -> (w1638:u8[])
                          n532 = call <userlib>:"LVClass_HasoSlopes Apply Substractor.vi"("HasoSlopes in"=w1623, "HasoSlopes to substract"=w1622, "error in (no error)"=w1626) -> ("HasoSlopes out"=w1627:refnum<class "HasoSlopes.lvclass">, "error out"=w1625:errorcluster)  [unwired: 11 in]
                          n533 = call "slopes2phase.vi"("TypePhase"=WavefrontReconstructionMode."Modal_Zernike", "Number of coefficients"=u8 32, "error in (no error)"=w1625, "Filter"=w1638, "HasoSlopes in"=w1627, "Phase in"=w1641) -> ("error out"=w1634:errorcluster, "HasoSlopes out"=w1635:refnum<class "HasoSlopes.lvclass">, "Phase out"=w1640:refnum<class "Phase.lvclass">)  [unwired: 3 in]
                          n534 = local read "idxType"() -> (w1629:enum16{"Wyant", "ANSI"})
                          n535 = call "slopes2zern.vi"("HasoSlopes in"=w1635, "error in (no error)"=w1634, "idxType"=w1629) -> ("HasoSlopes out"=w1624:refnum<class "HasoSlopes.lvclass">, "Zernike Coefficients"=w1628:dbl[], "error out"=w1633:errorcluster)  [unwired: 3 in, 2 out]
                          n536 = call <userlib>:"LVClass_Pupil ctor from HasoSlopes.vi"("Pupil in"=w1639, "HasoSlopes.lvclass"=w1627, "error in (no error)"=w1633) -> ("Pupil out"=w1649:refnum<class "Pupil.lvclass">, "error out"=w1650:errorcluster)  [unwired: 11 in]
                          n537 = case shown="True" w1632 {
                            tunnel: w1631 -> [_ w1660]
                            tunnel: w1630 -> [_ w1659]
                            tunnel: w1628 -> [_ w1658]
                            tunnel: w1627 -> [_ w1656]
                            tunnel: w1622 -> [_ w1657]
                            frame False {
                            }
                            frame True {
                              n538 = stacked-sequence {
                                tunnel: w1660 -> [w1664 w1671 w1677]
                                tunnel: w1659 -> [w1663 w1670 w1676]
                                tunnel: w1658 -> [_ _ w1675]
                                tunnel: w1657 -> [w1661 _ _]
                                tunnel: w1656 -> [_ w1668 _]
                                frame #0 {
                                n539 = Concatenate Strings(w1664, "_slopesOffset", ".has") -> (w1667:string)
                                n540 = Build Path(base path=w1663, name or relative path=w1667) -> (appended path=w1662:path)
                                n541 = call <userlib>:"LVClass_HasoSlopes Save.vi"("HasoSlopes in"=w1661, "path"=w1662) -> ()  [unwired: 12 in, 2 out]
                                }
                                frame #1 {
                                n542 = Concatenate Strings(w1671, "_slopesNet", ".has") -> (w1674:string)
                                n543 = Build Path(base path=w1670, name or relative path=w1674) -> (appended path=w1669:path)
                                n544 = call <userlib>:"LVClass_HasoSlopes Save.vi"("HasoSlopes in"=w1668, "path"=w1669) -> ()  [unwired: 12 in, 2 out]
                                }
                                frame #2 {
                                n545 = Concatenate Strings(w1677, "_zernCoefNet", ".txt") -> (w1680:string)
                                n546 = Build Path(base path=w1676, name or relative path=w1680) -> (appended path=w1681:path)
                                n547 = Array To Spreadsheet String(array=w1675, 3:"%f") -> (spreadsheet string=w1682:string)  [unwired: 1 in]
                                n548 = Write to Text File(file (use dialog)=w1681, text=w1682) -> ()  [unwired: 2 in, 3 out]
                                }
                              }
                            }
                          }
                          n549 = call <userlib>:"LVClasse_Phase GetStatisticDatas.vi"("Phase in"=w1640, "error in (no error)"=w1650) -> ("Phase out"=w1655:refnum<class "Phase.lvclass">, "StatisticsData"=w1636:T2, "error out"=w1653:errorcluster)  [unwired: 11 in]
                          n550 = local write "Phase statistics"(w1636) -> ()
                          n551 = call <userlib>:"LVClasse_Phase Get Data.vi"("Phase in"=w1655, "Pupil"=w1649, "error in (no error)"=w1653) -> ("Phase out"=w1651:refnum<class "Phase.lvclass">, "data"=w1637:sgl[][], "Pupil (dup)"=w1652:refnum<class "Pupil.lvclass">, "error out"=w1654:errorcluster)  [unwired: 9 in]
                          n552 = local write "Zernike Measured"(w1628) -> ()
                          n553 = local write "Phase values"(w1637) -> ()
                        }
                        frame Error {
                        }
                      }
                      n554 = call <userlib>:"LVClass_HasoSlopes dtor.vi"("HasoSlopes in"=w1575) -> ()  [unwired: 13 in, 2 out]
                    }
                  }
                }
              }
              n555 = Unbundle By Name(w1542) -> ("status"=w1543:bool)
            }
          }
        }
      }
      event "Exit": Value Change {
        # "STOP AND EXIT"
        n556 = event-data() -> ()  [unwired: 1 in, 4 out]
        n557 = case shown="False" w1708 {
          tunnel: w1716 -> [w1719 w1722]
          tunnel: [errorcluster {"status"=FALSE, "code"=0, "source"=""} ("error out") w1721] -> w1715
          tunnel: [w1719 w1720] -> w1714
          frame False {
          }
          frame True {
            n558 = call <userlib>:"LVClass_Camera stop acquisition.vi"("Camera in"=w1722) -> ("Camera out"=w1720:refnum<class "Camera.lvclass">, "error out"=w1721:errorcluster)  [unwired: 13 in]
          }
        }
      }
      event Panel Close? {
        n559 = event-data() -> ()  [unwired: 1 in, 1 out]
        n560 = flat-sequence {
          tunnel: w1738 -> [w1744]
          tunnel: w1731 -> [w1741]
          tunnel: [w1743] -> w1724
          tunnel: [w1742] -> w1723
          tunnel: [w1746] -> w1736
          tunnel: [w1747] -> w1737
          tunnel: w1724 -> [w1747]
          tunnel: w1723 -> [w1746]
          frame #0 {
            n561 = call <userlib>:"LVClass_Camera stop acquisition.vi"("Camera in"=w1744, "error in (no error)"=w1741) -> ("Camera out"=w1743:refnum<class "Camera.lvclass">, "error out"=w1742:errorcluster)  [unwired: 12 in]
          }
          frame #1 {
            n562 = local write "HASO ready"(FALSE) -> ()
          }
        }
        n563 = event-data("Discard?"=TRUE) -> ()  [unwired: 1 in, 1 out]
      }
    }
    n564 = Wait (ms)(milliseconds to wait=u32 250) -> ()  [unwired: 1 out]
  }
  n565 = case shown="True" w24 {
    tunnel: w46 -> [_ w1772]
    tunnel: w45 -> [_ w1771]
    tunnel: w44 -> [_ w1770]
    tunnel: w43 -> [_ w1769]
    tunnel: w42 -> [_ w1768]
    tunnel: w41 -> [_ w1767]
    tunnel: w40 -> [_ w1766]
    tunnel: w9 -> [_ w1759]
    tunnel: w5 -> [_ w1758]
    tunnel: w4 -> [_ w1757]
    tunnel: w3 -> [_ w1756]
    tunnel: w1 -> [_ w1753]
    tunnel: w2 -> [_ w1748]
    frame False {
    }
    frame True {
      n566 = flat-sequence {
        tunnel: w1771 -> [w1809]
        tunnel: w1772 -> [w1807]
        tunnel: [w1809] -> w1786
        tunnel: w1766 -> [w1808]
        tunnel: [w1808] -> w1785
        tunnel: [w1807] -> w1784
        tunnel: w1770 -> [w1806]
        tunnel: w1769 -> [w1805]
        tunnel: w1768 -> [w1804]
        tunnel: w1767 -> [w1803]
        tunnel: [w1802] -> w1783
        tunnel: [w1801] -> w1782
        tunnel: [w1800] -> w1781
        tunnel: [w1799] -> w1780
        tunnel: [w1792] -> w1764
        tunnel: [w1793] -> w1762
        tunnel: [w1794] -> w1760
        tunnel: w1759 -> [w1798]
        tunnel: w1758 -> [w1797]
        tunnel: w1757 -> [w1796]
        tunnel: w1756 -> [w1795]
        tunnel: [w1791] -> w1754
        tunnel: w1753 -> [w1790]
        tunnel: [w1789] -> w1752
        tunnel: w1748 -> [w1788]
        tunnel: [w1788] -> w1749
        tunnel: w1786 -> [w1824]
        tunnel: w1785 -> [w1823]
        tunnel: w1784 -> [w1821]
        tunnel: [w1823] -> w1779
        tunnel: [w1822] -> w1778
        tunnel: [w1821] -> w1777
        tunnel: w1783 -> [w1820]
        tunnel: [w1820] -> w1776
        tunnel: w1782 -> [w1819]
        tunnel: [w1819] -> w1775
        tunnel: w1781 -> [w1818]
        tunnel: [w1818] -> w1774
        tunnel: w1780 -> [w1817]
        tunnel: [w1817] -> w1773
        tunnel: [w1816] -> w1765
        tunnel: w1764 -> [w1816]
        tunnel: [w1815] -> w1763
        tunnel: w1762 -> [w1815]
        tunnel: [w1814] -> w1761
        tunnel: w1760 -> [w1814]
        tunnel: [w1813] -> w1755
        tunnel: w1754 -> [w1813]
        tunnel: w1752 -> [w1812]
        tunnel: [w1812] -> w1751
        tunnel: [w1811] -> w1750
        tunnel: w1749 -> [w1810]
        tunnel: w1779 -> [w1840]
        tunnel: w1778 -> [w1838]
        tunnel: w1777 -> [w1837]
        tunnel: w1776 -> [w1836]
        tunnel: w1775 -> [w1835]
        tunnel: w1774 -> [w1834]
        tunnel: w1773 -> [w1833]
        tunnel: w1765 -> [w1831]
        tunnel: w1763 -> [w1830]
        tunnel: w1761 -> [w1829]
        tunnel: w1755 -> [w1828]
        tunnel: w1751 -> [w1827]
        tunnel: w1750 -> [w1826]
        frame #0 {
          n567 = call <userlib>:"LVClass_Image dtor.vi"("Image in"=w1805) -> ("error out"=w1801:errorcluster)  [unwired: 13 in, 1 out]
          n568 = local write "HASO ready"(FALSE) -> ()
          n569 = call <userlib>:"LVClass_HasoSlopes dtor.vi"("HasoSlopes in"=w1798) -> ("error out"=w1793:errorcluster)  [unwired: 13 in, 1 out]
          n570 = call <userlib>:"LVClass_Pupil dtor.vi"("Pupil in"=w1795) -> ("error out"=w1791:errorcluster)  [unwired: 13 in, 1 out]
          n571 = call <userlib>:"LVClass_Image dtor.vi"("Image in"=w1803) -> ("error out"=w1799:errorcluster)  [unwired: 13 in, 1 out]
          n572 = call <userlib>:"LVClass_WavefrontCorrector dtor.vi"("WavefrontCorrector in"=w1790) -> ("error out"=w1789:errorcluster)  [unwired: 13 in, 1 out]
          n573 = call <userlib>:"LVClass_Image dtor.vi"("Image in"=w1806) -> ("error out"=w1802:errorcluster)  [unwired: 13 in, 1 out]
          n574 = call <userlib>:"LVClass_Image dtor.vi"("Image in"=w1804) -> ("error out"=w1800:errorcluster)  [unwired: 13 in, 1 out]
          n575 = call <userlib>:"LVClass_HasoEngine dtor.vi"("HasoEngine in"=w1796) -> ("error out"=w1792:errorcluster)  [unwired: 13 in, 1 out]
          n576 = call <userlib>:"LVClasse_Phase dtor.vi"("Phase in"=w1797) -> ("error out"=w1794:errorcluster)  [unwired: 13 in, 1 out]
        }
        frame #1 {
          n577 = call <userlib>:"LVClass_Camera dtor.vi"("Camera in"=w1824) -> ("error out"=w1822:errorcluster)  [unwired: 13 in, 1 out]
          n578 = call <userlib>:"LVClass_WavefrontCorrectorSet dtor.vi"("WavefrontCorrectorSet in"=w1810) -> ("error out"=w1811:errorcluster)  [unwired: 13 in, 1 out]
        }
        frame #2 {
          n579 = call <userlib>:"LVClass_CameraSet dtor.vi"("CameraSet.lvclass"=w1840) -> ("error out"=w1839:errorcluster)  [unwired: 13 in, 1 out]
          n580 = local write "Current status"("Shut down") -> ()
          n581 = Merge Errors(w1839, w1838, w1837, w1836, w1835, w1834, w1833, w1829, w1830, w1831, w1828, w1827, w1826) -> (w1832:errorcluster)
          n582 = property on="Current error" class="Clust (strict)"("Value"=w1832) -> ()  [unwired: 2 in, 2 out]
        }
      }
    }
  }
